vi "DDemo6_-G3.vi"() -> ()   [LabVIEW 2019]
uses:
  uStat400/DropSens uStat400 vis/Parameters.ctl
  uStat400/DropSens uStat400 vis/Serial - Settings mod.ctl
panel:
  out "position":bool
  out "main":bool
  out "graphs":bool
  out "potentiostat":bool
  in  "XI/YI":bool
  out "Camera":bool
  out "YV Graph":cluster{"X array":dbl[], "y array":dbl[]}(graph)
  out "XV Graph":cluster{"X array":dbl[], "y array":dbl[]}(graph)
  out "Iarray":dbl[](array[numeric])
  out "Yarray":dbl[](array[numeric])
  out "Xarray":dbl[](array[numeric])
  out "Moving":i32
  out "Status":bool
  out "error out":errorcluster
  out "Curves":cluster{dbl[], dbl[]}[](array[cluster])=[{[0.1, 0.102, 0.104, 0.106, 0.108, 0.11, 0.112, 0.114, 0.116, 0.118, 0.12, 0.122, 0.124, 0.126, 0.128, 0.13, 0.132, 0.134, 0.136, 0.138, 0.14, 0.142, 0.144, 0.146, 0.148, 0.15, 0.152, 0.154, 0.156, 0.158, 0.16, 0.162, 0.164, 0.166, 0.168, 0.17, 0.172, 0.174, 0.176, 0.178, 0.18, 0.182, 0.184, 0.186, 0.188, 0.19, 0.192, 0.194, 0.196, 0.198, 0.2, 0.202, 0.204, 0.206, 0.208, 0.21, 0.212, 0.214, 0.216, 0.218, 0.22, 0.222, 0.224, 0.226, 0.228, 0.23, 0.232, 0.234, 0.236, 0.238, 0.24, 0.242, 0.244, 0.246, 0.248, 0.25, 0.252, 0.254, 0.256, 0.258, 0.26, 0.262, 0.264, 0.266, 0.268, 0.27, 0.272, 0.274, 0.276, 0.278, 0.28, 0.282, 0.284, 0.286, 0.288, 0.29, 0.292, 0.294, 0.296, 0.298, 0.3, 0.302, 0.304, 0.306, 0.308, 0.31, 0.312, 0.314, 0.316, 0.318, 0.32, 0.322, 0.324, 0.326, 0.328, 0.33, 0.332, 0.334, 0.336, 0.338, 0.34, 0.342, 0.344, 0.346, 0.348, 0.35, 0.352, 0.354, 0.356, 0.358, 0.36, 0.362, 0.364, 0.366, 0.368, 0.37, 0.372, 0.374, 0.376, 0.378, 0.38, 0.382, 0.384, 0.386, 0.388, 0.39, 0.392, 0.394, 0.396, 0.398, 0.4, 0.402, 0.404, 0.406, 0.408, 0.41, 0.412, 0.414, 0.416, 0.418, 0.42, 0.422, 0.424, 0.426, 0.428, 0.43, 0.432, 0.434, 0.436, 0.438, 0.44, 0.442, 0.444, 0.446, 0.448, 0.45, 0.452, 0.454, 0.456, 0.458, 0.46, 0.462, 0.464, 0.466, 0.468, 0.47, 0.472, 0.474, 0.476, 0.478, 0.48, 0.482, 0.484, 0.486, 0.488, 0.49, 0.492, 0.494, 0.496, 0.498, 0.5, 0.502, 0.504, 0.506, 0.508, 0.51, 0.512, 0.514, 0.516, 0.518, 0.52, 0.522, 0.524, 0.526, 0.528, 0.53, 0.532, 0.534, 0.536, 0.538, 0.54, 0.542, 0.544, 0.546, 0.548, 0.55, 0.552, 0.554, 0.556, 0.558, 0.56, 0.562, 0.564, 0.566, 0.568, 0.57, 0.572, 0.574, 0.576, 0.578, 0.58, 0.582, 0.584, 0.586, 0.588, 0.59, 0.592, 0.594, 0.596, 0.598, 0.6, 0.602, 0.604, 0.606, 0.608, 0.61, 0.612, 0.614, 0.616, 0.618, 0.62, 0.622, 0.624, 0.626, 0.628, 0.63, 0.632, 0.634, 0.636, 0.638, 0.64, 0.642, 0.644, 0.646, 0.648, 0.65, 0.652, 0.654, 0.656, 0.658, 0.66, 0.662, 0.664, 0.666, 0.668, 0.67, 0.672, 0.674, 0.676, 0.678, 0.68, 0.682, 0.684, 0.686, 0.688, 0.69, 0.692, 0.694, 0.696, 0.698, 0.7, 0.702, 0.704, 0.706, 0.708, 0.71, 0.712, 0.714, 0.716, 0.718, 0.72, 0.722, 0.724, 0.726, 0.728, 0.73, 0.732, 0.734, 0.736, 0.738, 0.74, 0.742, 0.744, 0.746, 0.748, 0.75, 0.752, 0.754, 0.756, 0.758, 0.76, 0.762, 0.764, 0.766, 0.768, 0.77, 0.772, 0.774, 0.776, 0.778, 0.78, 0.782, 0.784, 0.786, 0.788, 0.79, 0.792, 0.794, 0.796, 0.798, 0.8, 0.802, 0.804, 0.806, 0.808, 0.81, 0.812, 0.814, 0.816, 0.818, 0.82, 0.822, 0.824, 0.826, 0.828, 0.83, 0.832, 0.834, 0.836, 0.838, 0.84, 0.842, 0.844, 0.846, 0.848, 0.85, 0.852, 0.854, 0.856, 0.858, 0.86, 0.862, 0.864, 0.866, 0.868, 0.87, 0.872, 0.874, 0.876, 0.878, 0.88, 0.882, 0.884, 0.886, 0.888, 0.89, 0.892, 0.894, 0.896, 0.898, 0.9], [5e-05, 6.25e-05, 5e-05, 6.25e-05, 5e-05, 5e-05, 5e-05, 7.5e-05, 5e-05, 6.25e-05, 5e-05, 6.25e-05, 5e-05, 6.25e-05, 5e-05, 6.25e-05, 5e-05, 6.25e-05, 5e-05, 6.25e-05, 5e-05, 6.25e-05, 5e-05, 6.25e-05, 5e-05, 6.25e-05, 5e-05, 6.25e-05, 3.75e-05, 7.5e-05, 5e-05, 6.25e-05, 5e-05, 6.25e-05, 5e-05, 6.25e-05, 5e-05, 6.25e-05, 5e-05, 6.25e-05, 5e-05, 7.5e-05, 5e-05, 6.25e-05, 5e-05, 6.25e-05, 5e-05, 7.5e-05, 6.25e-05, 6.25e-05, 5e-05, 6.25e-05, 5e-05, 7.5e-05, 5e-05, 6.25e-05, 5e-05, 6.25e-05, 5e-05, 6.25e-05, 5e-05, 6.25e-05, 5e-05, 7.5e-05, 5e-05, 6.25e-05, 5e-05, 7.5e-05, 6.25e-05, 6.25e-05, 5e-05, 6.25e-05, 5e-05, 6.25e-05, 5e-05, 6.25e-05, 5e-05, 6.25e-05, 5e-05, 6.25e-05, 5e-05, 6.25e-05, 5e-05, 6.25e-05, 5e-05, 6.25e-05, 5e-05, 6.25e-05, 5e-05, 6.25e-05, 5e-05, 6.25e-05, 5e-05, 6.25e-05, 5e-05, 6.25e-05, 5e-05, 6.25e-05, 3.75e-05, 6.25e-05, 5e-05, 6.25e-05, 5e-05, 6.25e-05, 5e-05, 6.25e-05, 5e-05, 6.25e-05, 5e-05, 6.25e-05, 5e-05, 6.25e-05, 5e-05, 6.25e-05, 5e-05, 7.5e-05, 5e-05, 7.5e-05, 5e-05, 6.25e-05, 5e-05, 6.25e-05, 5e-05, 7.5e-05, 3.75e-05, 6.25e-05, 5e-05, 7.5e-05, 5e-05, 7.5e-05, 3.75e-05, 7.5e-05, 5e-05, 6.25e-05, 5e-05, 7.5e-05, 5e-05, 6.25e-05, 5e-05, 7.5e-05, 3.75e-05, 7.5e-05, 5e-05, 6.25e-05, 5e-05, 6.25e-05, 5e-05, 6.25e-05, 5e-05, 7.5e-05, 3.75e-05, 7.5e-05, 3.75e-05, 6.25e-05, 5e-05, 6.25e-05, 5e-05, 7.5e-05, 3.75e-05, 6.25e-05, 5e-05, 6.25e-05, 5e-05, 6.25e-05, 3.75e-05, 7.5e-05, 5e-05, 7.5e-05, 3.75e-05, 6.25e-05, 5e-05, 6.25e-05, 3.75e-05, 6.25e-05, 5e-05, 6.25e-05, 5e-05, 6.25e-05, 5e-05, 6.25e-05, 5e-05, 7.5e-05, 5e-05, 7.5e-05, 5e-05, 6.25e-05, 5e-05, 7.5e-05, 5e-05, 7.5e-05, 5e-05, 7.5e-05, 5e-05, 7.5e-05, 5e-05, 7.5e-05, 5e-05, 7.5e-05, 6.25e-05, 8.75e-05, 6.25e-05, 7.5e-05, 5e-05, 7.5e-05, 5e-05, 7.5e-05, 5e-05, 7.5e-05, 6.25e-05, 7.5e-05, 5e-05, 7.5e-05, 5e-05, 7.5e-05, 5e-05, 7.5e-05, 5e-05, 7.5e-05, 5e-05, 6.25e-05, 5e-05, 7.5e-05, 5e-05, 7.5e-05, 5e-05, 6.25e-05, 5e-05, 7.5e-05, 3.75e-05, 6.25e-05, 3.75e-05, 6.25e-05, 3.75e-05, 6.25e-05, 3.75e-05, 6.25e-05, 5e-05, 7.5e-05, 5e-05, 7.5e-05, 5e-05, 7.5e-05, 3.75e-05, 7.5e-05, 5e-05, 7.5e-05, 5e-05, 6.25e-05, 3.75e-05, 6.25e-05, 5e-05, 6.25e-05, 3.75e-05, 7.5e-05, 5e-05, 6.25e-05, 3.75e-05, 6.25e-05, 5e-05, 6.25e-05, 5e-05, 6.25e-05, 5e-05, 7.5e-05, 3.75e-05, 6.25e-05, 5e-05, 6.25e-05, 3.75e-05, 7.5e-05, 5e-05, 6.25e-05, 5e-05, 6.25e-05, 5e-05, 6.25e-05, 5e-05, 6.25e-05, 5e-05, 6.25e-05, 5e-05, 6.25e-05, 3.75e-05, 6.25e-05, 5e-05, 6.25e-05, 5e-05, 7.5e-05, 5e-05, 6.25e-05, 5e-05, 6.25e-05, 5e-05, 6.25e-05, 5e-05, 6.25e-05, 5e-05, 6.25e-05, 3.75e-05, 6.25e-05, 3.75e-05, 6.25e-05, 5e-05, 6.25e-05, 3.75e-05, 6.25e-05, 3.75e-05, 6.25e-05, 5e-05, 6.25e-05, 5e-05, 6.25e-05, 5e-05, 6.25e-05, 5e-05, 6.25e-05, 5e-05, 6.25e-05, 5e-05, 7.5e-05, 5e-05, 6.25e-05, 3.75e-05, 6.25e-05, 5e-05, 7.5e-05, 5e-05, 7.5e-05, 5e-05, 6.25e-05, 5e-05, 7.5e-05, 3.75e-05, 6.25e-05, 5e-05, 7.5e-05, 5e-05, 6.25e-05, 5e-05, 6.25e-05, 5e-05, 7.5e-05, 3.75e-05, 6.25e-05, 5e-05, 6.25e-05, 5e-05, 7.5e-05, 5e-05, 6.25e-05, 5e-05, 6.25e-05, 3.75e-05, 6.25e-05, 3.75e-05, 6.25e-05, 3.75e-05, 7.5e-05, 3.75e-05, 6.25e-05, 5e-05, 6.25e-05, 3.75e-05, 6.25e-05, 3.75e-05, 6.25e-05, 5e-05, 7.5e-05, 5e-05, 6.25e-05, 5e-05, 6.25e-05, 3.75e-05, 6.25e-05, 3.75e-05, 6.25e-05, 5e-05, 5e-05, 3.75e-05, 6.25e-05, 5e-05, 6.25e-05, 3.75e-05, 6.25e-05, 3.75e-05, 6.25e-05, 5e-05, 6.25e-05, 3.75e-05, 6.25e-05, 3.75e-05, 7.5e-05, 3.75e-05, 6.25e-05, 5e-05, 6.25e-05, 5e-05, 6.25e-05, 5e-05, 6.25e-05, 5e-05]}, ...(4 in all)]
  in  "Serial Settings":T1={"baud rate"=115200, "data bits"=8, "parity"=enum."None", "stop bits"=10, "flow control"=0} {"flow control" items=["None"=0, "XON/XOFF"=1, "RTS/CTS"=2, "DTR/DSR"=4]; "stop bits" items=["1.0"=10, "1.5"=15, "2.0"=20]; "data bits" min=5 max=8 step=1; "baud rate" items=["75"=75, "110"=110, "134"=134, "150"=150, "300"=300, "600"=600, "1200"=1200, "1800"=1800, "2400"=2400, "4800"=4800, "7200"=7200, "9600"=9600, "14400"=14400, "19200"=19200, "28800"=28800, "38400"=38400, "56000"=56000, "57600"=57600, "115200"=115200, "128000"=128000, "230400"=230400]}
  in  "Node list":string[](tree)=["Node 1 - Ch1"]
  in  "Cluster 5":T3={"Parameters M"=[{"Param"="Estep [V]", "Values"=0.002}, {"Param"="Srate [V/s]", "Values"=0.05}], "Parameters N 8"=[], "Parameters N 7"=[], "Parameters N 6"=[], "Parameters N 5"=[{"Param"="Ebegin [V]", "Values"=0.1}, {"Param"="Eend [V]", "Values"=0.9}, {"Param"="Estep [V]", "Values"=0.002}, {"Param"="Srate [V/s]", "Values"=0.05}], "Parameters N 4"=[{"Param"="Ebegin [V]", "Values"=0.1}, {"Param"="Eend [V]", "Values"=0.9}], "Parameters N 3"=[{"Param"="Ebegin [V]", "Values"=0.1}, {"Param"="Eend [V]", "Values"=0.9}], "Parameters N 2"=[{"Param"="Ebegin [V]", "Values"=0.1}, {"Param"="Eend [V]", "Values"=0.9}], "Parameters N 1"=[{"Param"="Ebegin [V]", "Values"=0.1}, {"Param"="Eend [V]", "Values"=0.9}, {"Param"="Estep [V]", "Values"=0.002}, {"Param"="Srate [V/s]", "Values"=0.05}]}
  in  "Cluster 4":T4={"Pretr M"=[{"Param"="Econd [V]", "Values"=0.0}, {"Param"="Tcond [s]", "Values"=0.0}, {"Param"="Edep [V]", "Values"=0.0}, {"Param"="Tdep [s]", "Values"=0.0}, {"Param"="Tequil [s]", "Values"=3.0}], "Pretr N 7"=[{"Param"="Econd [V]", "Values"=0.0}, {"Param"="Tcond [s]", "Values"=0.0}, {"Param"="Edep [V]", "Values"=0.0}, {"Param"="Tdep [s]", "Values"=0.0}, {"Param"="Tequil [s]", "Values"=3.0}], "Pretr N 5"=[{"Param"="Econd [V]", "Values"=0.0}, {"Param"="Tcond [s]", "Values"=0.0}, {"Param"="Edep [V]", "Values"=0.0}, {"Param"="Tdep [s]", "Values"=0.0}, {"Param"="Tequil [s]", "Values"=3.0}], "Pretr N 4"=[{"Param"="Econd [V]", "Values"=0.0}, {"Param"="Tcond [s]", "Values"=0.0}, {"Param"="Edep [V]", "Values"=0.0}, {"Param"="Tdep [s]", "Values"=0.0}, {"Param"="Tequil [s]", "Values"=3.0}], "Pretr N 3"=[{"Param"="Econd [V]", "Values"=0.0}, {"Param"="Tcond [s]", "Values"=0.0}, {"Param"="Edep [V]", "Values"=0.0}, {"Param"="Tdep [s]", "Values"=0.0}, {"Param"="Tequil [s]", "Values"=3.0}], "Pretr N 2"=[{"Param"="Econd [V]", "Values"=0.0}, {"Param"="Tcond [s]", "Values"=0.0}, {"Param"="Edep [V]", "Values"=0.0}, {"Param"="Tdep [s]", "Values"=0.0}, {"Param"="Tequil [s]", "Values"=3.0}], "Pretr N 1"=[{"Param"="Econd [V]", "Values"=0.0}, {"Param"="Tcond [s]", "Values"=0.0}, {"Param"="Edep [V]", "Values"=0.0}, {"Param"="Tdep [s]", "Values"=0.0}, {"Param"="Tequil [s]", "Values"=3.0}], "Pretr N 8"=[{"Param"="Econd [V]", "Values"=0.0}, {"Param"="Tcond [s]", "Values"=0.0}, {"Param"="Edep [V]", "Values"=0.0}, {"Param"="Tdep [s]", "Values"=0.0}, {"Param"="Tequil [s]", "Values"=3.0}], "Pretr N 6"=[{"Param"="Econd [V]", "Values"=0.0}, {"Param"="Tcond [s]", "Values"=0.0}, {"Param"="Edep [V]", "Values"=0.0}, {"Param"="Tdep [s]", "Values"=0.0}, {"Param"="Tequil [s]", "Values"=3.0}]}
  in  "Cluster 3":T5 {"Option N 1"."StandbyPot" format="%.3g"; "Option N 2"."StandbyPot" format="%.3g"; "Option N 4"."StandbyPot" format="%.3g"; "Option N 6"."StandbyPot" format="%.3g"; "Option N 7"."StandbyPot" format="%.3g"; "Option N 8"."StandbyPot" format="%.3g"; "Option N 3"."StandbyPot" format="%.3g"; "Option N 5"."StandbyPot" format="%.3g"; "Option M"."StandbyPot" format="%.3g"}
  in  "Cluster 2":T6
  out "Cluster":T7={"Technique M"="Linear Sweep Voltammetry", "Technique N 8"="Linear Sweep Voltammetry", "Technique N 7"="Linear Sweep Voltammetry", "Technique N 6"="Linear Sweep Voltammetry", "Technique N 5"="Linear Sweep Voltammetry", "Technique N 4"="Linear Sweep Voltammetry", "Technique N 3"="Linear Sweep Voltammetry", "Technique N 2"="Linear Sweep Voltammetry", "Technique N 1"="Linear Sweep Voltammetry"}
  in  "XYXA":bool
  out "Image Out":T8(plugin-control)
  out "ArAy":string[](array[string])
  out "ArAx":string[](array[string])
  out "Rel_act_pos":string
  out "True A":dbl format="%#.3g"
  out "True Z":dbl format="%#.3f"
  out "True Y":dbl format="%#.3f"
  out "True X":dbl format="%#.3f"
  out "MDI":string
  in  "Tab Control":T9(tab)
  in  "Copy current position":bool
  in  "Stop all":bool
  in  "Move":bool
  in  "A":dbl
  in  "Z":dbl
  in  "Y":dbl
  in  "X":dbl
  in  "Home":bool
  out "Sent value":string
  in  "A-":bool
  in  "A+":bool
  in  "stop step":bool
  in  "z-":bool
  in  "z+":bool
  out "Step":bool
  out "Jog":bool=TRUE
  in  "Step size (mm)":dbl
  in  "Jog?":bool=TRUE
  in  "Speed (mm/s) manual":dbl(knob)=10.0 min=1.0 max=500.0 step=1.0 scale=1.0..500.0 scale format="%#_6f"
  in  "y-":bool
  in  "y+":bool
  in  "x-":bool
  in  "x+":bool
  out "manual":bool
  in  "2D stop":bool
  in  "Wait (ms)":dbl=1.0 min=1.0 step=1.0
  in  "Speed (micron/s) 2D":dbl(knob)=1.0 min=1.0 max=500.0 step=1.0 scale=1.0..500.0 scale format="%#_6f"
  in  "2D start":bool
  in  "No. of teps":dbl=1.0 min=1.0 step=1.0
  in  "Y1":dbl step=0.0001 format="%#.3f"
  in  "Y0":dbl step=0.0001 format="%#.3f"
  in  "X1":dbl step=0.001 format="%#.3f"
  in  "X0":dbl step=0.001 format="%#.3f"
  in  "Stop A":bool
  out "String":string
  in  "Speed (micron/s) A":dbl(knob)=1.0 min=1.0 max=500.0 step=1.0 scale=1.0..500.0 scale format="%#_6f"
  in  "y0":dbl min=0.0 step=0.001 format="%#.3f"
  in  "x0":dbl min=0.0 step=0.001 format="%#.3f"
  in  "x1":dbl min=0.0 step=0.001 format="%#.3f"
  in  "y1":dbl min=0.0 step=0.001 format="%#.3f"
  in  "Line displacement":dbl=0.001 min=0.001 step=0.001 format="%#_3f"
  in  "Step size":dbl=0.001 min=0.001 step=0.001 format="%#_3f"
  in  "Area start":bool
  in  "Wait (ms) Area":dbl=1000.0 min=1.0 step=1.0
  out "Status":bool
  out "Actual I/U 2":dbl
  out "Config Status":u8(slide)=73 scale=0.0..66.0
  out "Actual Values":T10 {"Actual I/U" format="%#_6f"}
  in  "VISA resource name":refnum<visa-resource-name>="COM5"
  in  "Check port":bool
  in  "stop Measuring":bool
  out "result":bool
  # "Target position"
  # "Start"
  # "Finish"
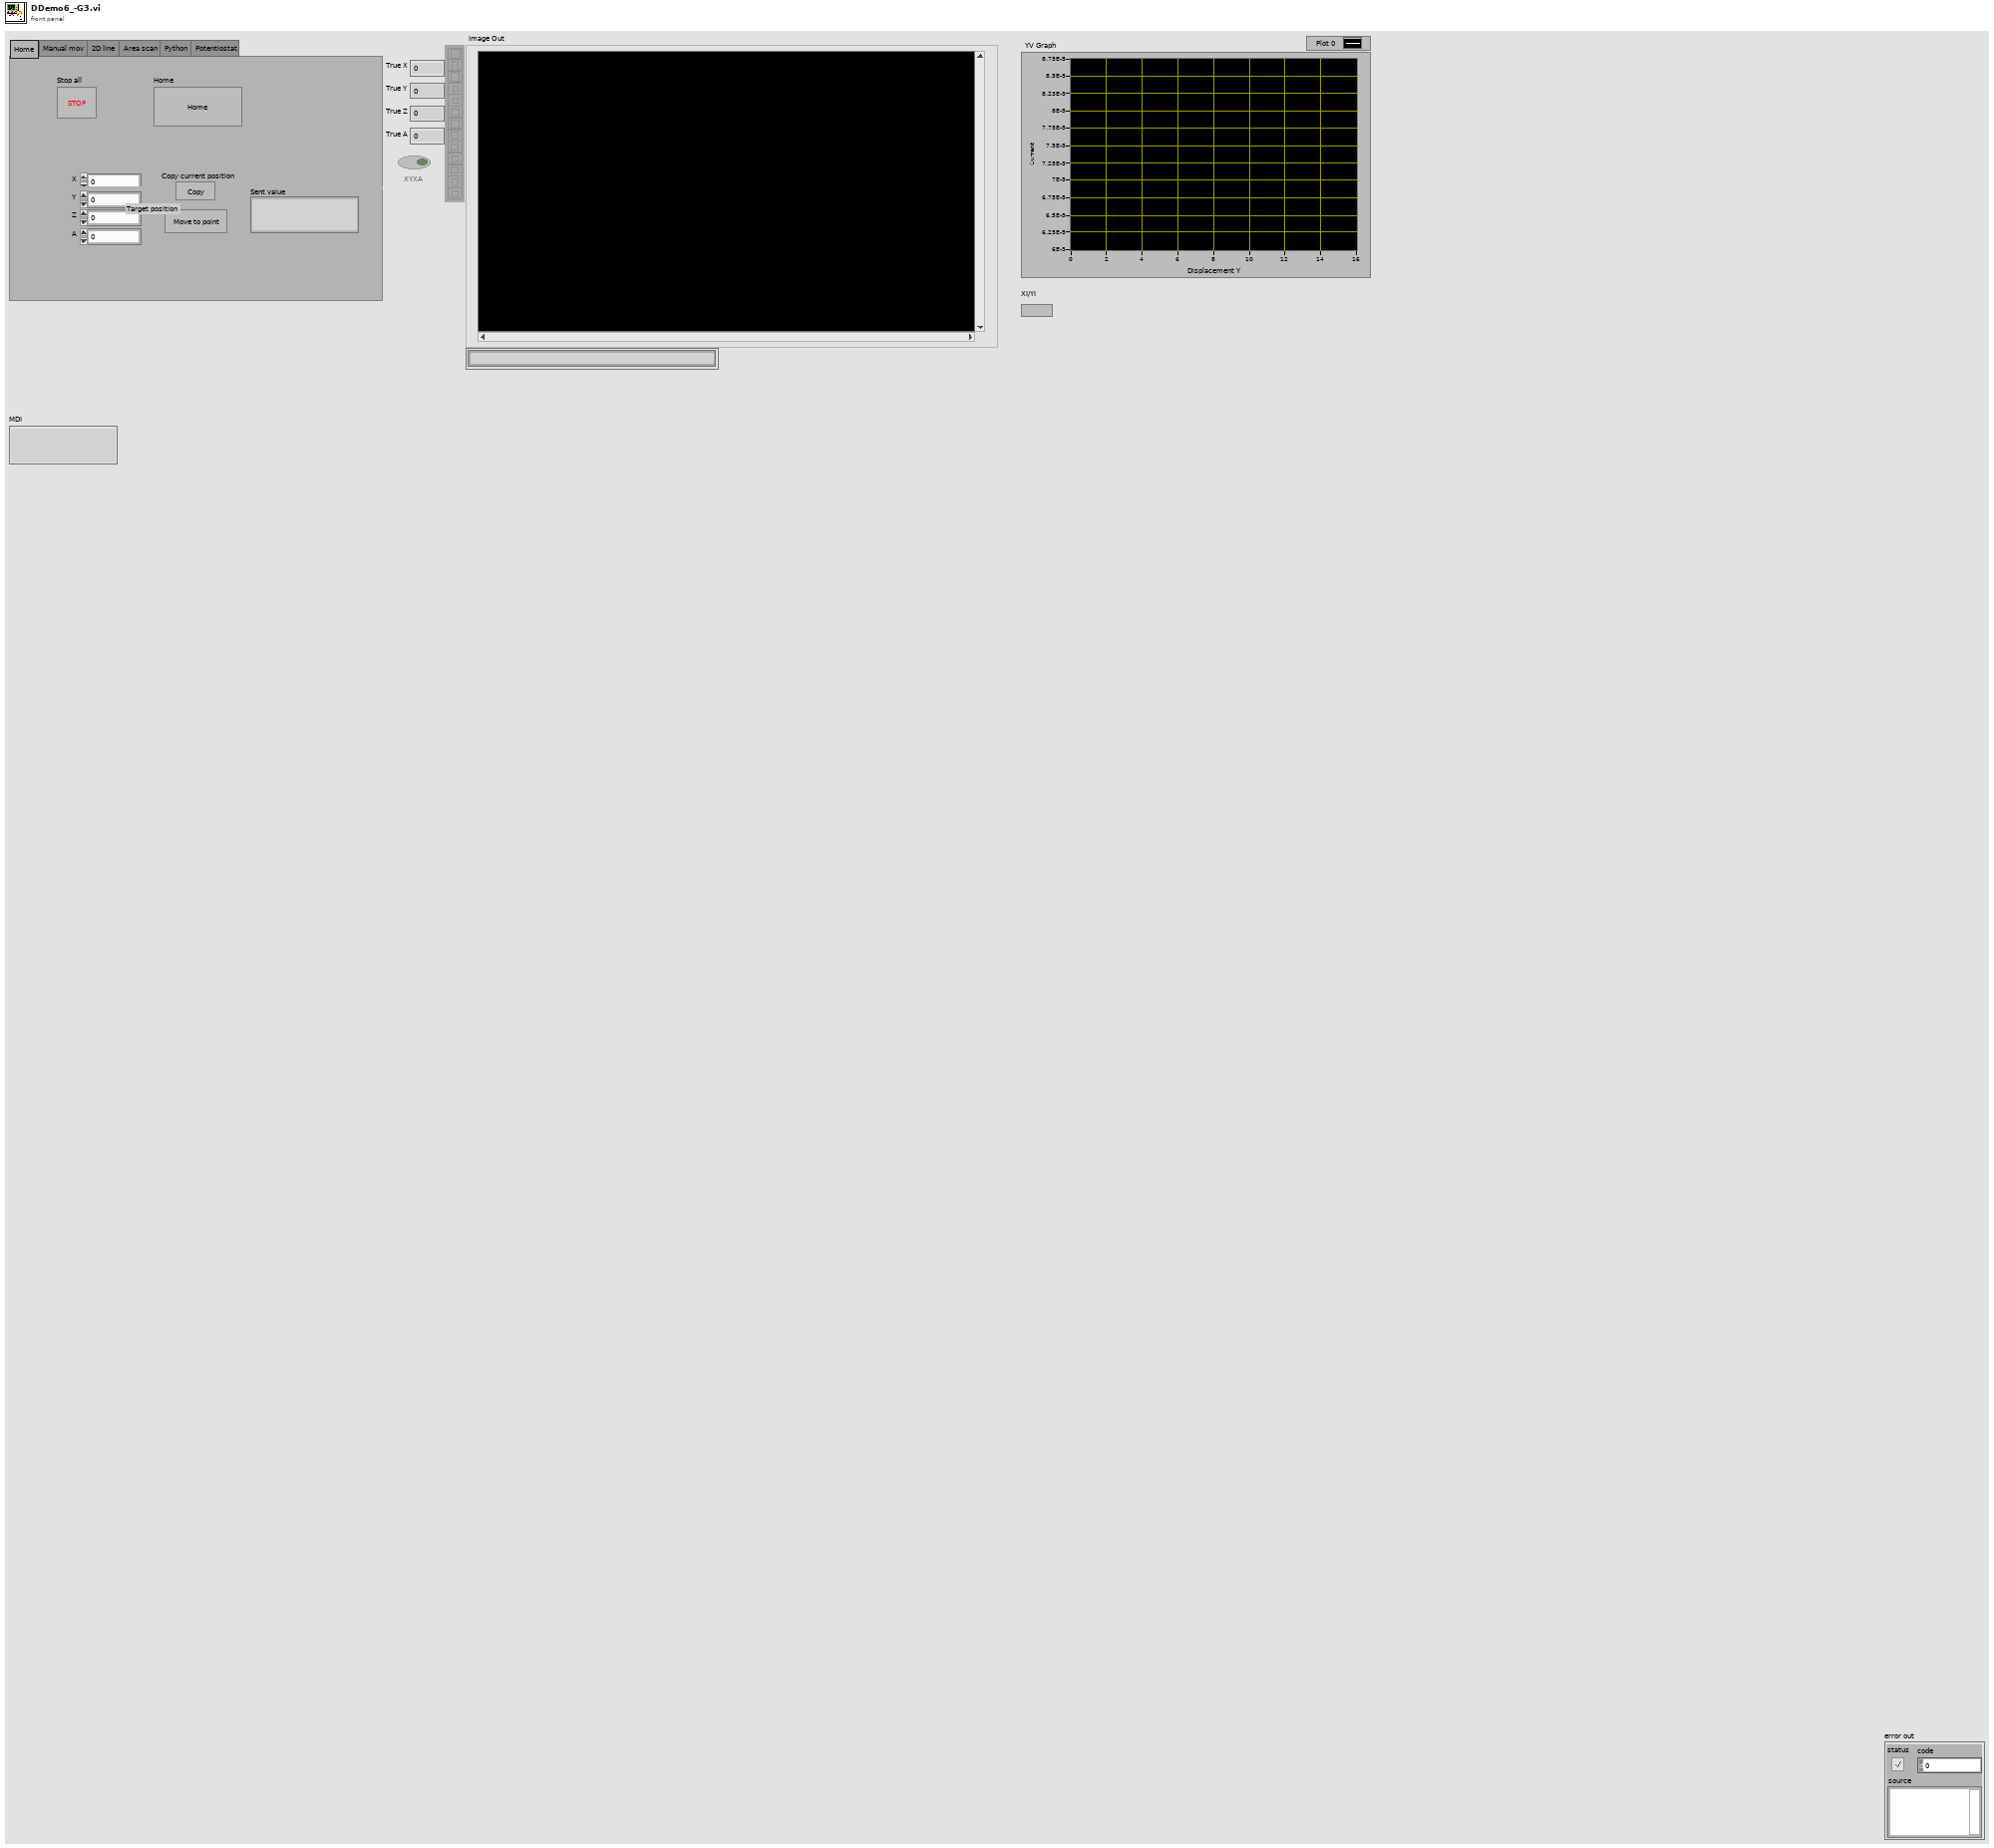
[diagram p1: front panel]
types:
  T1 = typedef "Serial - Settings mod.ctl" = cluster{"baud rate":u32, "data bits":u16, "parity":enum16{"None", "Odd", "Even", "Mark", "Space"}, "stop bits":u16, "flow control":u16}
  T2 = typedef "Parameters.ctl" = cluster{"Param":string, "Values":dbl}[]
  T3 = cluster{"Parameters M":T2, "Parameters N 8":T2, "Parameters N 7":T2, "Parameters N 6":T2, "Parameters N 5":T2, "Parameters N 4":T2, "Parameters N 3":T2, "Parameters N 2":T2, "Parameters N 1":T2}
  T4 = cluster{"Pretr M":T2, "Pretr N 7":T2, "Pretr N 5":T2, "Pretr N 4":T2, "Pretr N 3":T2, "Pretr N 2":T2, "Pretr N 1":T2, "Pretr N 8":T2, "Pretr N 6":T2}
  T5 = cluster{"Option M":cluster{"Cells":enum32{"No Selection", "Leave cell on", "Standby potential"}, "StandbyPot":dbl}, "Option N 5":cluster{"Cells":enum32{"No Selection", "Leave cell on", "Standby potential"}, "StandbyPot":dbl}, "Option N 3":cluster{"Cells":enum32{"No Selection", "Leave cell on", "Standby potential"}, "StandbyPot":dbl}, "Option N 8":cluster{"Cells":enum32{"No Selection", "Leave cell on", "Standby potential"}, "StandbyPot":dbl}, "Option N 7":cluster{"Cells":enum32{"No Selection", "Leave cell on", "Standby potential"}, "StandbyPot":dbl}, "Option N 6":cluster{"Cells":enum32{"No Selection", "Leave cell on", "Standby potential"}, "StandbyPot":dbl}, "Option N 4":cluster{"Cells":enum32{"No Selection", "Leave cell on", "Standby potential"}, "StandbyPot":dbl}, "Option N 2":cluster{"Cells":enum32{"No Selection", "Leave cell on", "Standby potential"}, "StandbyPot":dbl}, "Option N 1":cluster{"Cells":enum32{"No Selection", "Leave cell on", "Standby potential"}, "StandbyPot":dbl}}
  T6 = cluster{"CR N 8":enum16{"Auto", "10 mA", "1 mA", "100 uA", "10 uA", "1 uA", "100 nA", "10 nA", "1 nA"}, "CR N 7":enum16{"Auto", "10 mA", "1 mA", "100 uA", "10 uA", "1 uA", "100 nA", "10 nA", "1 nA"}, "CR N 6":enum16{"Auto", "10 mA", "1 mA", "100 uA", "10 uA", "1 uA", "100 nA", "10 nA", "1 nA"}, "CR N 5":enum16{"Auto", "10 mA", "1 mA", "100 uA", "10 uA", "1 uA", "100 nA", "10 nA", "1 nA"}, "CR N 4":enum16{"Auto", "10 mA", "1 mA", "100 uA", "10 uA", "1 uA", "100 nA", "10 nA", "1 nA"}, "CR N 3":enum16{"Auto", "10 mA", "1 mA", "100 uA", "10 uA", "1 uA", "100 nA", "10 nA", "1 nA"}, "CR N 2":enum16{"Auto", "10 mA", "1 mA", "100 uA", "10 uA", "1 uA", "100 nA", "10 nA", "1 nA"}, "CR N 1":enum16{"Auto", "10 mA", "1 mA", "100 uA", "10 uA", "1 uA", "100 nA", "10 nA", "1 nA"}}
  T7 = cluster{"Technique M":string, "Technique N 8":string, "Technique N 7":string, "Technique N 6":string, "Technique N 5":string, "Technique N 4":string, "Technique N 3":string, "Technique N 2":string, "Technique N 1":string}
  T8 = typedef "IMAQ Image.ctl" = refnum<image>
  T9 = enum32{"Home", "Manual mov", "2D line", "Area scan", "Python", "Potentiostat"}
  T10 = cluster{"Actual I/U":dbl, "Actual V/T":dbl, "No of Ch":i16}
  T11 = enum16{"Main", "Line", "Area Move", "Enable all", "Move to target", "Get Values"}
  T12 = typedef "Comunication.ctl" = cluster{"VISA resource name out":refnum<visa-resource-name>, "Techniques":T13[], "Tree 2":refnum<vi>, "Nodes":i32[], "Radio Buttons":enum32{"M 1x8", "M 8x1"}, "queue ref":refnum<queue>}
  T13 = typedef "Techniques.ctl" = enum16{"Linear Sweep Voltammetry", "Cyclic Voltammetry", "Square Wave Voltammetry", "Differential Pulse Voltammetry", "Normal Pulse Voltammetry", "Normal Dif. Pulse Voltametry", "AC Voltametry", "Linear Polarization Resistance", "LSV+AD", "CV+AD", "Amperometric Detection", "Zero Resistance Amperometry", "Fast Amperometry", "Pulsed Amperometric Detection", "Multipulsed Amperometric Detection", "Coulometric Detection", "Linear Sweep Potentiometry", "Cyclic Potentiometry", "Potentiometric Detection", "Zero Current Potentiometry", "Fast Potentiometry", "Multipulsed Potentiometric Detection", "PSA Faradaic", "PSA Galvanostatic"}
  T14 = enum8{"Enabled", "Disabled", "Disabled and Grayed Out"}
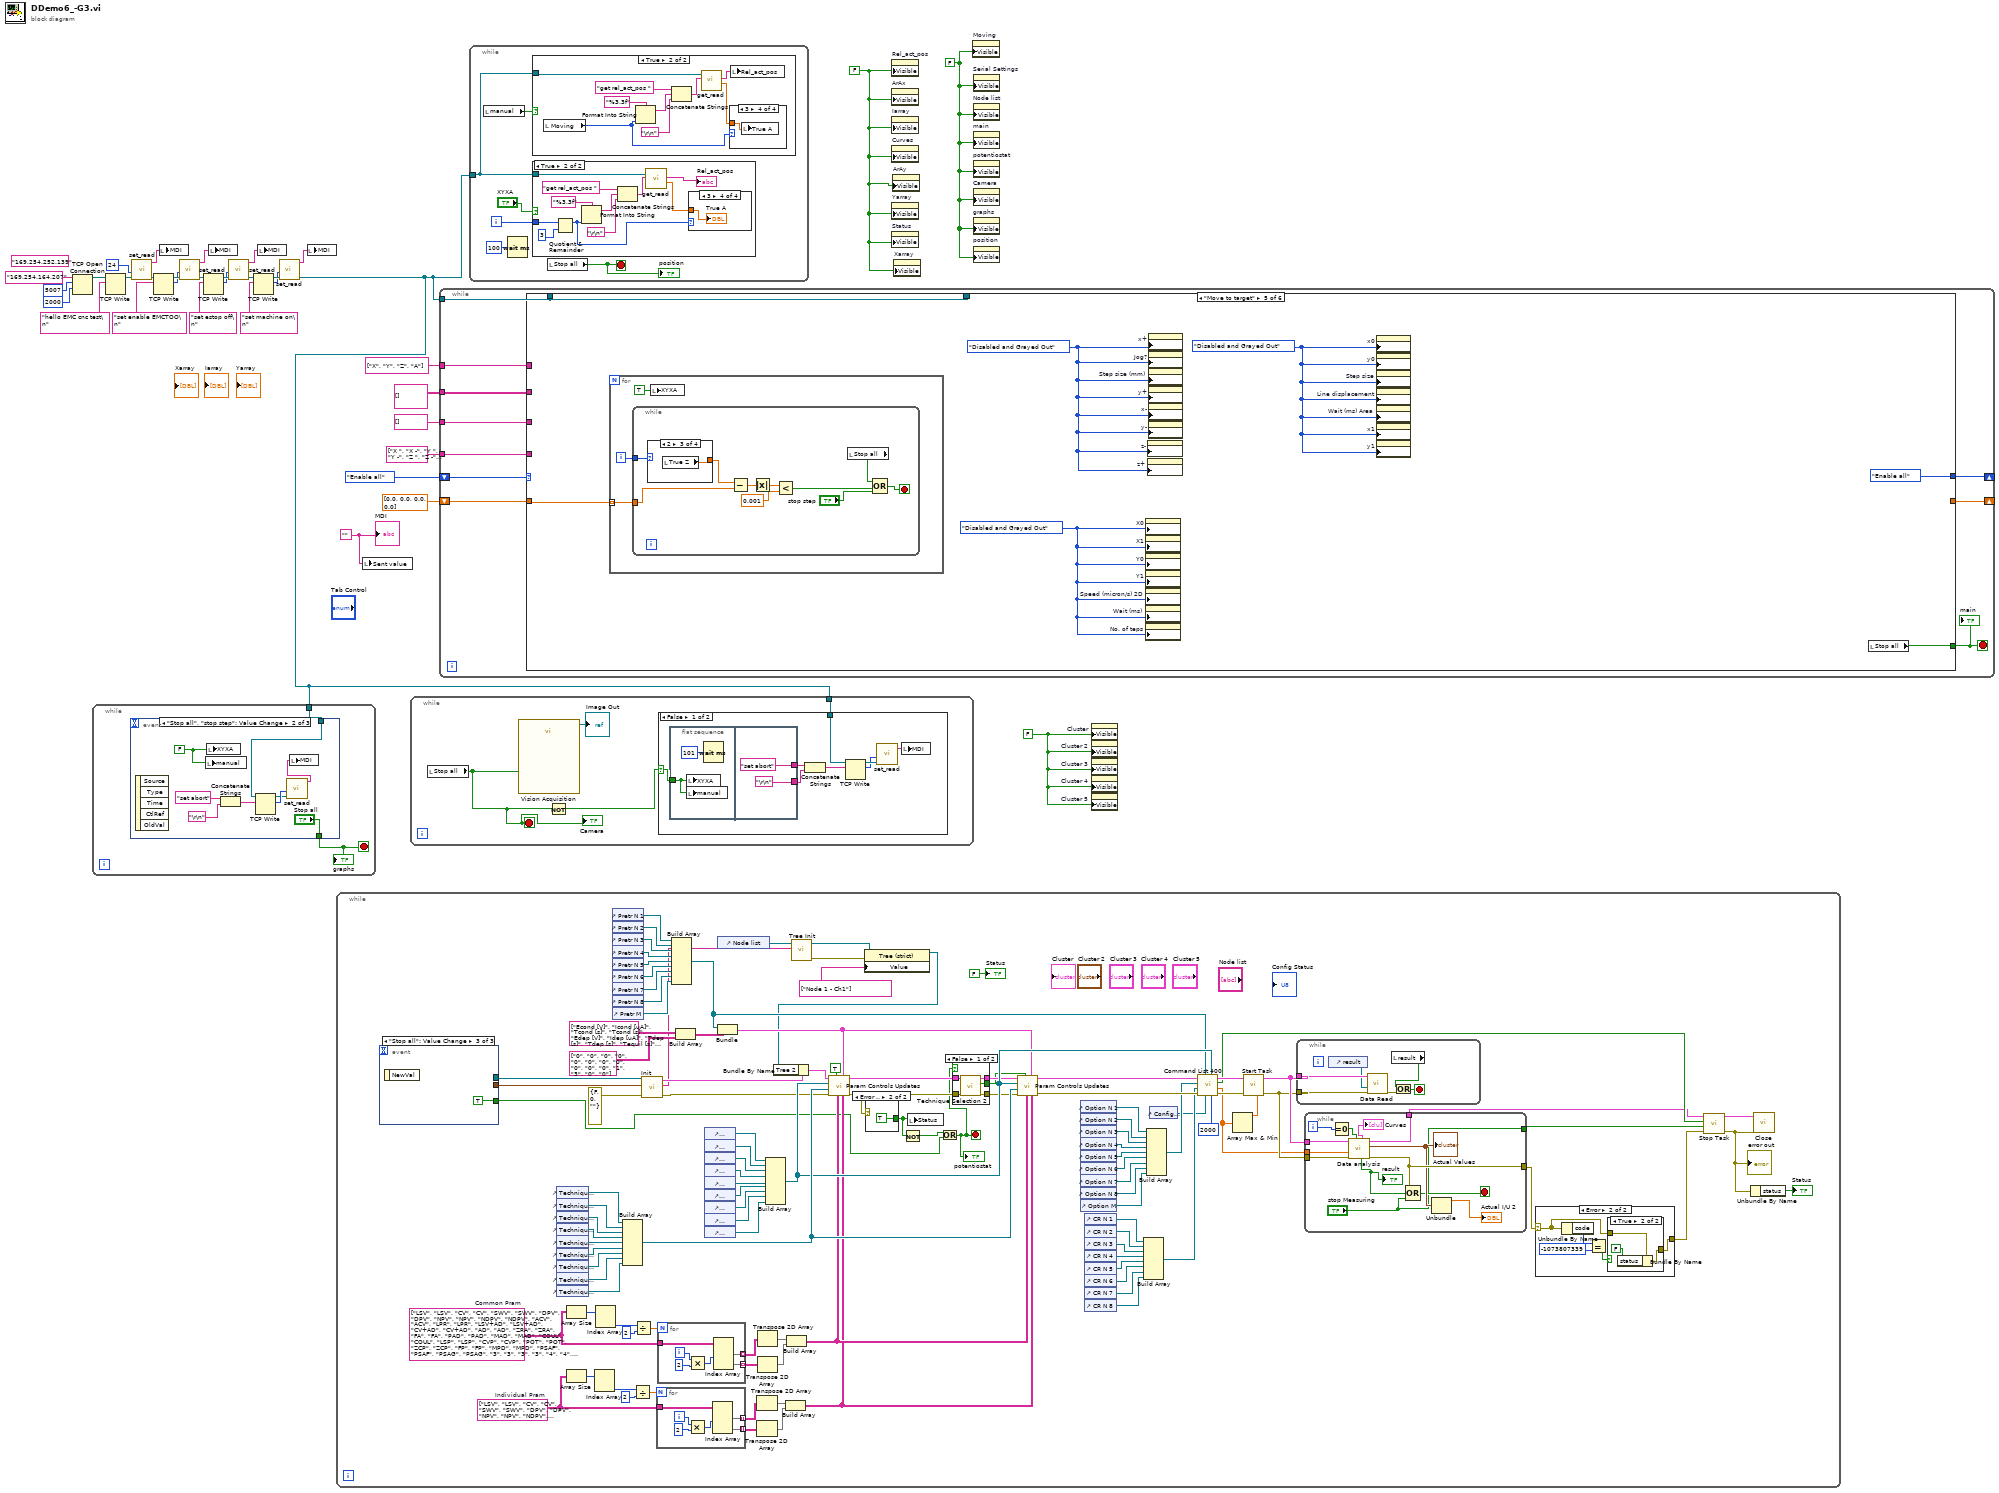
[diagram p0: block diagram]
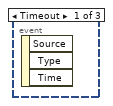
[diagram p3: hidden frame]
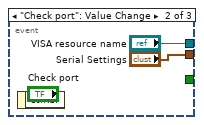
[diagram p4: hidden frame]
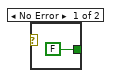
[diagram p5: hidden frame]
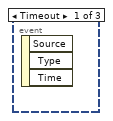
[diagram p8: hidden frame]
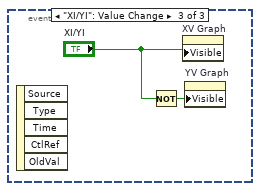
[diagram p9: hidden frame]
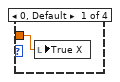
[diagram p12: hidden frame]
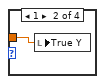
[diagram p13: hidden frame]
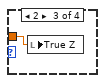
[diagram p14: hidden frame]
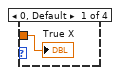
[diagram p16: hidden frame]
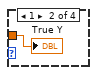
[diagram p17: hidden frame]
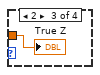
[diagram p18: hidden frame]
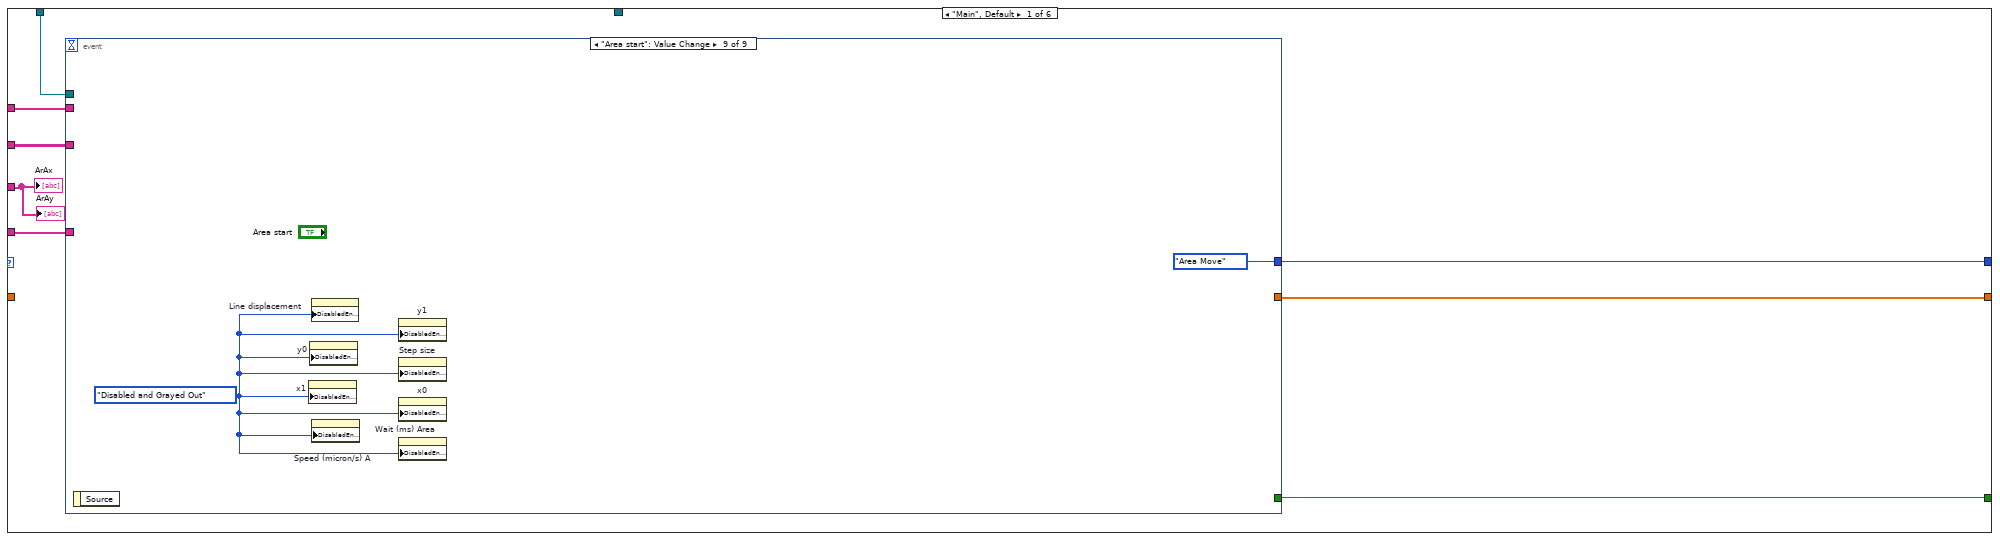
[diagram p19: hidden frame]
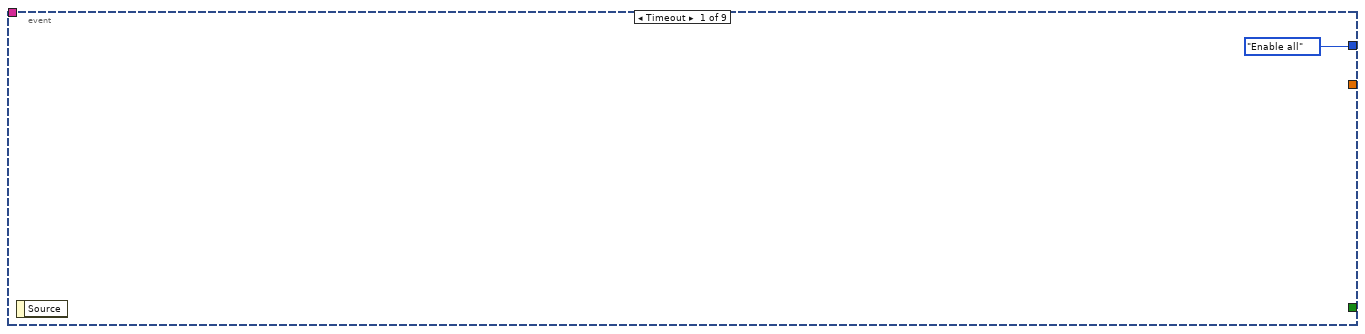
[diagram p20: hidden frame]
diagram:
  w1 = FALSE
  w2 = FALSE
  w5 = FALSE ("Visible")
  (unwired) "169.254.252.139"
  w32 = ""
  n1 = TCP Open Connection(address="169.254.164.207", remote port or service name=5007, timeout ms (60000)=2000) -> (connection ID=w28:refnum<k5>)  [unwired: 2 in, 1 out]
  n2 = TCP Write(connection ID=w28, data in="hello EMC cnc test\n") -> (connection ID out=w27:refnum<k5>)  [unwired: 2 in, 2 out]
  n3 = call "set_read.vi"("connection ID"=w27, "bytes to read"=24) -> ("connection ID 2"=w26:refnum<k5>, "concatenated string"=w13:string)  [unwired: 4 in]
  n4 = TCP Write(connection ID=w26, data in="set enable EMCTOO\n") -> (connection ID out=w25:refnum<k5>, bytes written=w12:i32)  [unwired: 2 in, 1 out]
  n5 = local write "MDI"(w13) -> ()
  n6 = call "set_read.vi"("connection ID"=w25, "bytes to read"=w12) -> ("connection ID 2"=w24:refnum<k5>, "concatenated string"=w16:string)  [unwired: 4 in]
  n7 = TCP Write(connection ID=w24, data in="set estop off\n") -> (connection ID out=w23:refnum<k5>, bytes written=w11:i32)  [unwired: 2 in, 1 out]
  n8 = local write "MDI"(w16) -> ()
  n9 = call "set_read.vi"("connection ID"=w23, "bytes to read"=w11) -> ("connection ID 2"=w22:refnum<k5>, "concatenated string"=w15:string)  [unwired: 4 in]
  n10 = TCP Write(connection ID=w22, data in="set machine on\n") -> (connection ID out=w21:refnum<k5>, bytes written=w10:i32)  [unwired: 2 in, 1 out]
  n11 = local write "MDI"(w15) -> ()
  n12 = call "set_read.vi"("connection ID"=w21, "bytes to read"=w10) -> ("connection ID 2"=w3:refnum<k5>, "concatenated string"=w14:string)  [unwired: 4 in]
  n13 = while {
    tunnel: w3 -> [w36]
    stop <- w35 stop-if-true
    n14 = event shown="[1] \"Stop all\", \"stop step\": Value Change" {
      selector: _ -> [_ _ _]
      dyn-events: _ -> [_ _ _]
      timeout: _ -> [_ _ _]
      tunnel: w36 -> [_ w42 _]
      tunnel: [_ "Stop all" _] -> w35
      event Timeout {
        n15 = event-data() -> ()  [unwired: 1 in, 3 out]
      }
      event "Stop all", "stop step": Value Change {
        w45 = FALSE
        n16 = event-data() -> ()  [unwired: 1 in, 5 out]
        n17 = local write "manual"(w45) -> ()
        n18 = local write "XYXA"(w45) -> ()
        n19 = Concatenate Strings("set abort", "\r\n") -> (w39:string)
        n20 = TCP Write(connection ID=w42, data in=w39) -> (connection ID out=w43:refnum<k5>, bytes written=w44:i32)  [unwired: 2 in, 1 out]
        n21 = call "set_read.vi"("connection ID"=w43, "bytes to read"=w44) -> ("concatenated string"=w38:string)  [unwired: 4 in, 1 out]
        n22 = local write "MDI"(w38) -> ()
      }
      event "XI/YI": Value Change {
        n23 = event-data() -> ()  [unwired: 1 in, 5 out]
        n24 = Not(x="XI/YI") -> (.not. x?=w47:bool)
        n25 = property on="XV Graph" class="XYGraph (strict)"("Visible"="XI/YI") -> ()  [unwired: 2 in, 2 out]
        n26 = property on="YV Graph" class="XYGraph (strict)"("Visible"=w47) -> ()  [unwired: 2 in, 2 out]
      }
    }
    "graphs" <- w35
  }
  n27 = local write "MDI"(w14) -> ()
  n28 = while {
    stop <- w48 stop-if-true
    w58 = string[][] [["LSV", "LSV", "CV", "CV", "SWV", "SWV", "DPV", "DPV", "NPV", "NPV", "NDPV", "NDPV", "ACV", "ACV", "LPR", "LPR", "LSV+AD", "LSV+AD", "CV+AD", "CV+AD", "AD", "AD", "ZRA", "ZRA", "FA", "FA", "PAD", "PAD", "MAD", "MAD", "COUL", "COUL", "LSP", "LSP", "CVP", "CVP", "POT", "POT", "ZCP", "ZCP", "FP", "FP", "MPD", "MPD", "PSAF", "PSAF", "PSAG", "PSAG"], ["2", "2", "3", "3", "2", "2", "2", "2", "2", "2", "2", "2", "2", "2", "2", "2", "0", "0", "0", "0", "1", "1", "0", "0", "1", "1", "1", "1", "8", "8", "1", "1", "2", "2", "3", "3", "1", "1", "0", "0", "1", "1", "8", "8", "0", "0", "0", "0"], ["Ebegin [V]", "0.1", "Ebegin [V]", "0.1", "Ebegin [V]", "0.45", "Ebegin [V]", "0.45", "Ebegin [V]", "0", "Ebegin [V]", "0", "Ebegin [V]", "-0.9", "Ebegin [V]", "-0.1", "", "", "", "", "E [V]", "-0.1", "", "", "E [V]", "-0.1", "Ei [V]", "-0.1", "Steps", "1", "E [V]", "-0.1", "Ibegin [uA]", "0", "Ibegin [uA]", "0.5", "Ibegin [uA]", "-5", "", "", "Ibegin [uA]", "0", "Steps", "1", "", "", "", ""], ["Eend [V]", "0.9", "Evtx1 [V]", "0.9", "Eend [V]", "-0.15", "Eend [V]", "-0.15", "Eend [V]", "0.5", "Eend [V]", "0.5", "Eend [V]", "-0.2", "Eend [V]", "0.1", "", "", "", "", "", "", "", "", "", "", "", "", "Cell off", "1", "", "", "Iend [uA]", "0.5", "Ivtx1 [uA]", "1", "", "", "", "", "", "", "Cell off", "1", "", "", "", ""], ["", "", "Evtx2 [V]", "-0.1", "", "", "", "", "", "", "", "", "", "", "", "", "", "", "", "", "", "", "", "", "", "", "", "", "Limits", "1", "", "", "", "", "Ivtx2 [uA]", "0", "", "", "", "", "", "", "Limits", "1", "", "", "", ""], ["", "", "", "", "", "", "", "", "", "", "", "", "", "", "", "", "", "", "", "", "", "", "", "", "", "", "", "", "Cell 1 [Off/On]", "1", "", "", "", "", "", "", "", "", "", "", "", "", "Cell 1 [Off/On]", "1", "", "", "", ""], ["", "", "", "", "", "", "", "", "", "", "", "", "", "", "", "", "", "", "", "", "", "", "", "", "", "", "", "", "E1 [V]", "0.1", "", "", "", "", "", "", "", "", "", "", "", "", "I1 [uA]", "100", "", "", "", ""], ["", "", "", "", "", "", "", "", "", "", "", "", "", "", "", "", "", "", "", "", "", "", "", "", "", "", "", "", "t1 [s]", "1", "", "", "", "", "", "", "", "", "", "", "", "", "t1 [s]", "1", "", "", "", ""], ["", "", "", "", "", "", "", "", "", "", "", "", "", "", "", "", "", "", "", "", "", "", "", "", "", "", "", "", "Lim1> [uA]", "40000", "", "", "", "", "", "", "", "", "", "", "", "", "Lim1> [V]", "4.095", "", "", "", ""], ["", "", "", "", "", "", "", "", "", "", "", "", "", "", "", "", "", "", "", "", "", "", "", "", "", "", "", "", "Lim1< [uA]", "-40000", "", "", "", "", "", "", "", "", "", "", "", "", "Lim< [V]", "-4.095", "", "", "", ""], ["", "", "", "", "", "", "", "", "", "", "", "", "", "", "", "", "", "", "", "", "", "", "", "", "", "", "", "", "", "", "", "", "", "", "", "", "", "", "", "", "", "", "", "", "", "", "", ""], ["", "", "", "", "", "", "", "", "", "", "", "", "", "", "", "", "", "", "", "", "", "", "", "", "", "", "", "", "", "", "", "", "", "", "", "", "", "", "", "", "", "", "", "", "", "", "", ""], ["", "", "", "", "", "", "", "", "", "", "", "", "", "", "", "", "", "", "", "", "", "", "", "", "", "", "", "", "", "", "", "", "", "", "", "", "", "", "", "", "", "", "", "", "", "", "", ""], ["", "", "", "", "", "", "", "", "", "", "", "", "", "", "", "", "", "", "", "", "", "", "", "", "", "", "", "", "", "", "", "", "", "", "", "", "", "", "", "", "", "", "", "", "", "", "", ""], ["", "", "", "", "", "", "", "", "", "", "", "", "", "", "", "", "", "", "", "", "", "", "", "", "", "", "", "", "", "", "", "", "", "", "", "", "", "", "", "", "", "", "", "", "", "", "", ""]]  # Individual Pram
    w59 = string[][] [["LSV", "LSV", "CV", "CV", "SWV", "SWV", "DPV", "DPV", "NPV", "NPV", "NDPV", "NDPV", "ACV", "ACV", "LPR", "LPR", "LSV+AD", "LSV+AD", "CV+AD", "CV+AD", "AD", "AD", "ZRA", "ZRA", "FA", "FA", "PAD", "PAD", "MAD", "MAD", "COUL", "COUL", "LSP", "LSP", "CVP", "CVP", "POT", "POT", "ZCP", "ZCP", "FP", "FP", "MPD", "MPD", "PSAF", "PSAF", "PSAG", "PSAG"], ["3", "3", "3", "3", "4", "4", "5", "5", "5", "5", "7", "7", "6", "6", "6", "6", "6", "6", "7", "7", "2", "2", "2", "2", "2", "2", "12", "12", "2", "2", "2", "2", "3", "3", "3", "3", "2", "2", "2", "2", "2", "2", "2", "2", "2", "2", "3", "3"], ["Estep [V]", "0.002", "Estep [V]", "0.002", "Estep [V]", "0.005", "Estep [V]", "0.004 [V]", "Estep [V]", "0.005", "Estep [V]", "0.005 [V]", "Estep [V]", "0.008", "dE/dt lim [uV/s]", "1", "Ebegin [V]", "0.1", "Ebegin [V]", "0.1", "Interval [s]", "0.1", "Interval [s]", "0.5", "Interval [ms]", "50", "E1 [V]", "0.4", "Interval [s]", "0.1", "Interval [s]", "0.5", "Istep [uA]", "0.005", "Istep [uA]", "0.01", "Interval [s]", "0.5", "Interval [s]", "0.5", "Interval [ms]", "10", "Internal [s]", "0.1", "Elimit [V]", "1", "Elimit [V]", "1"], ["Srate [V/s]", "0.05", "Srate [V/s]", "0.05", "Eamp [V]", "0.002", "Epuls [V]", "0.002", "Ebase [V]", "0", "tint [ms]", "50", "Eamp [V]", "0.1", "tmaxOCP [s]", "120", "Eend [V]", "0.9", "Evtx1 [V]", "0.9", "t [s]", "3600", "t [s]", "20", "t [s]", "20", "t1 [s]", "0.1", "Repeat [times]", "1", "t[s]", "30", "Srate [uA/s]", "0.2", "Srate [uA/s]", "0.1", "t [s]", "60", "t [s]", "60", "t [s]", "5", "Repeat [times]", "1", "tmax [s]", "10", "S.Cur [uA]", "10"], ["nscans", "1", "nscans", "1", "Freq [Hz]", "20", "tpuls [ms]", "10", "tmod [ms]", "25", "Ebase [V]", "0", "tmod [ms]", "160", "tprecond [s]", "5", "E2 [V]", "1", "Evtx2 [V]", "-0.1", "", "", "", "", "", "", "E2 [V]", "-0.2", "", "", "", "", "Nscans", "1", "Nscans", "1", "", "", "", "", "", "", "", "", "", "", "tmax [s]", "10"], ["", "", "", "", "nscans", "1", "Srate [V/s]", "0.04", "tint [ms]", "100", "Epuls [V]", "0.003", "Freq [Hz]", "50", "Estep [V]", "0.001", "Estep [V]", "0.002", "E2 [V]", "0.1", "", "", "", "", "", "", "t2 [s]", "0.2", "", "", "", "", "", "", "", "", "", "", "", "", "", "", "", "", "", "", "", ""], ["", "", "", "", "", "", "nscans", "1", "nscans", "1", "tpuls [ms]", "10", "tint [ms]", "560 [ms]", "Srate [V/s]", "0.001", "Srate [V/s]", "0.05", "Estep [V]", "0.002", "", "", "", "", "", "", "E3 [V]", "0.41", "", "", "", "", "", "", "", "", "", "", "", "", "", "", "", "", "", "", "", ""], ["", "", "", "", "", "", "", "", "", "", "tmod [ms]", "10", "nscans", "1", "nscans", "1", "nscans", "1", "Srate [V/s]", "0.05", "", "", "", "", "", "", "t3 [s]", "0.1", "", "", "", "", "", "", "", "", "", "", "", "", "", "", "", "", "", "", "", ""], ["", "", "", "", "", "", "", "", "", "", "nscans", "1", "", "", "", "", "", "", "nscans", "1", "", "", "", "", "", "", "E4 [V]", "-0.2", "", "", "", "", "", "", "", "", "", "", "", "", "", "", "", "", "", "", "", ""], ["", "", "", "", "", "", "", "", "", "", "", "", "", "", "", "", "", "", "", "", "", "", "", "", "", "", "t4 [s]", "0.2", "", "", "", "", "", "", "", "", "", "", "", "", "", "", "", "", "", "", "", ""], ["", "", "", "", "", "", "", "", "", "", "", "", "", "", "", "", "", "", "", "", "", "", "", "", "", "", "E5 [V]", "0.4", "", "", "", "", "", "", "", "", "", "", "", "", "", "", "", "", "", "", "", ""], ["", "", "", "", "", "", "", "", "", "", "", "", "", "", "", "", "", "", "", "", "", "", "", "", "", "", "t5 [s]", "0.1", "", "", "", "", "", "", "", "", "", "", "", "", "", "", "", "", "", "", "", ""], ["", "", "", "", "", "", "", "", "", "", "", "", "", "", "", "", "", "", "", "", "", "", "", "", "", "", "ti [s]", "0.3", "", "", "", "", "", "", "", "", "", "", "", "", "", "", "", "", "", "", "", ""], ["", "", "", "", "", "", "", "", "", "", "", "", "", "", "", "", "", "", "", "", "", "", "", "", "", "", "t [s]", "20", "", "", "", "", "", "", "", "", "", "", "", "", "", "", "", "", "", "", "", ""]]  # Common Pram
    n29 = event shown="[2] \"Stop all\": Value Change" {
      selector: _ -> [_ _ _]
      dyn-events: _ -> [_ _ _]
      timeout: _ -> [_ _ _]
      tunnel: [_ "VISA resource name" _] -> w52
      tunnel: [_ "Serial Settings" _] -> w51
      tunnel: [_ _ TRUE] -> w49
      event Timeout {
        n30 = event-data() -> ()  [unwired: 1 in, 3 out]
      }
      event "Check port": Value Change {
        n31 = event-data() -> ()  [unwired: 1 in, 1 out]
      }
      event "Stop all": Value Change {
        n32 = event-data() -> ()  [unwired: 1 in, 1 out]
      }
    }
    n33 = control-ref of="Technique N 1"() -> (w85:refnum<vi>)
    n34 = control-ref of="Technique N 2"() -> (w84:refnum<vi>)
    n35 = control-ref of="Technique N 3"() -> (w83:refnum<vi>)
    n36 = control-ref of="Technique N 4"() -> (w82:refnum<vi>)
    n37 = control-ref of="Technique N 5"() -> (w81:refnum<vi>)
    n38 = control-ref of="Technique N 6"() -> (w80:refnum<vi>)
    n39 = control-ref of="Technique N 7"() -> (w79:refnum<vi>)
    n40 = control-ref of="Technique N 8"() -> (w78:refnum<vi>)
    n41 = control-ref of="Technique M"() -> (w77:refnum<vi>)
    n42 = Array Size(array=w58) -> (size(s)=w60:i32[])
    n43 = Array Size(array=w59) -> (size(s)=w68:i32[])
    n44 = Index Array(array=w60) -> (element #2=w61:i32)  [unwired: 2 in, 1 out]
    n45 = Index Array(array=w68) -> (element #2=w69:i32)  [unwired: 2 in, 1 out]
    n46 = control-ref of="Pretr N 1"() -> (w109:refnum<vi>)
    n47 = control-ref of="Pretr N 2"() -> (w108:refnum<vi>)
    n48 = control-ref of="Pretr N 3"() -> (w107:refnum<vi>)
    n49 = control-ref of="Pretr N 4"() -> (w106:refnum<vi>)
    n50 = control-ref of="Pretr N 5"() -> (w105:refnum<vi>)
    n51 = control-ref of="Pretr N 6"() -> (w104:refnum<vi>)
    n52 = control-ref of="Pretr N 7"() -> (w103:refnum<vi>)
    n53 = control-ref of="Pretr N 8"() -> (w102:refnum<vi>)
    n54 = control-ref of="Pretr M"() -> (w101:refnum<vi>)
    n55 = Build Array(w85, w84, w83, w82, w81, w80, w79, w78, w77) -> (w158:refnum<vi>[])
    n56 = Divide(x=w61, y=2) -> (x/y=w63:dbl)
    n57 = Divide(x=w69, y=2) -> (x/y=w71:dbl)
    n58 = call "Init.vi"("error in"=errorcluster {"status"=FALSE, "code"=0, "source"=""}, "Serial Settings"=w51, "VISA Refnum in"=w52) -> ("error out"=w54:errorcluster, "Device model"=w55:string, "Cluster"=w56:T12)  [unwired: 6 in]
    n59 = for {
      N: w63 -> [_]
      tunnel: w58 -> [w180]
      tunnel: [w176] -> w64 mode=indexing
      tunnel: [w175] -> w65 mode=indexing
      i -> [w179]
      n60 = Multiply(x=w179, y=2) -> (x*y=w178:i32)
      n61 = Index Array(array=w180, index (col) #1=w178) -> (element #1=w176:string[], element #2=w175:string[])  [unwired: 3 in]
    }
    n62 = for {
      N: w71 -> [_]
      tunnel: w59 -> [w186]
      tunnel: [w182] -> w72 mode=indexing
      tunnel: [w181] -> w73 mode=indexing
      i -> [w185]
      n63 = Multiply(x=w185, y=2) -> (x*y=w184:i32)
      n64 = Index Array(array=w186, index (col) #1=w184) -> (element #1=w182:string[], element #2=w181:string[])  [unwired: 3 in]
    }
    n65 = Build Array(w109, w108, w107, w106, w105, w104, w103, w102, w101) -> (w156:refnum<vi>[])
    n66 = Build Array(string[][] [["Econd [V]", "Icond [uA]"], ["Tcond [s]", "Tcond [s]"], ["Edep [V]", "Idep [uA]"], ["Tdep [s]", "Tdep [s]"], ["Tequil [s]", "Tequil [s]"]], string[][] [["0", "0", "0"], ["0", "0", "0"], ["0", "0", "0"], ["0", "0", "1"], ["3", "0", "0"]]) -> (w110:string[][][])
    n67 = control-ref of="Parameters N 1"() -> (w87:refnum<vi>)
    n68 = control-ref of="Parameters N 2"() -> (w88:refnum<vi>)
    n69 = control-ref of="Parameters N 3"() -> (w89:refnum<vi>)
    n70 = control-ref of="Parameters N 4"() -> (w90:refnum<vi>)
    n71 = control-ref of="Parameters N 5"() -> (w91:refnum<vi>)
    n72 = control-ref of="Parameters N 6"() -> (w92:refnum<vi>)
    n73 = control-ref of="Parameters N 7"() -> (w86:refnum<vi>)
    n74 = control-ref of="Parameters N 8"() -> (w93:refnum<vi>)
    n75 = control-ref of="Parameters M"() -> (w94:refnum<vi>)
    n76 = control-ref of="Node list"() -> (w98:refnum<vi>)
    n77 = Bundle(w156, w110) -> (w155:cluster{refnum<vi>[], string[][][]})  [unwired: 1 in]
    n78 = Transpose 2D Array(2D array=w64) -> (transposed array=w66:string[][])
    n79 = Transpose 2D Array(2D array=w65) -> (transposed array=w67:string[][])
    n80 = Transpose 2D Array(2D array=w72) -> (transposed array=w74:string[][])
    n81 = Transpose 2D Array(2D array=w73) -> (transposed array=w75:string[][])
    n82 = Build Array(w87, w88, w89, w90, w91, w92, w86, w93, w94) -> (w157:refnum<vi>[])
    n83 = Build Array(w66, w67) -> (w153:string[][][])
    n84 = Build Array(w74, w75) -> (w154:string[][][])
    n85 = call "Tree Init.vi"("Model"=w55, "TreeControl in"=w98) -> ("error out"=w100:errorcluster, "TreeControl out"=w99:refnum<vi>)  [unwired: 8 in]
    n86 = property class="Tree (strict)"(reference=w99, error in=w100, "Value"=string[] ["Node 1 - Ch1"]) -> (reference out=w76:refnum<vi>)  [unwired: 1 out]
    n87 = Bundle By Name(cluster=w56, "Tree 2"=w76) -> (w96:T12)
    n88 = call "Param Controls Updates.vi"("Individual Pram"=w153, "Pretreatment"=w155, "Common Pram"=w154, "Accept St"=TRUE, "error in (no error)"=w54, "Technique"=w158, "Parameters"=w157, "Reference in"=w96) -> ("error out"=w160:errorcluster, "Reference out"=w159:T12)  [unwired: 2 in]
    n89 = case shown="Error .." w160 {
      tunnel: [FALSE TRUE] -> w57
      frame No Error {
      }
      frame Error {
      }
    }
    n90 = Not(x=w57) -> (.not. x?=w50:bool)
    n91 = local write "Status"(w57) -> ()
    n92 = Or(x=w50, y=w49) -> (x .or. y?=w48:bool)
    "potentiostat" <- w48
    n93 = case shown="False" w48 {
      selector: w48 -> [_ w167]
      tunnel: w160 -> [w166 w169]
      tunnel: w159 -> [w165 w168]
      tunnel: [w164 w169] -> w152
      tunnel: [w163 w168] -> w149
      tunnel: [w162 w167] -> w115
      frame False {
        n94 = call "Technique Selection 2.vi"("error in (no error)"=w166, "Reference In"=w165) -> ("error out"=w164:errorcluster, "Accept St"=w162:bool, "Reference Out"=w163:T12)  [unwired: 5 in, 2 out]
      }
      frame True {
      }
    }
    n95 = call "Param Controls Updates.vi"("Individual Pram"=w153, "Pretreatment"=w155, "Common Pram"=w154, "Accept St"=w115, "error in (no error)"=w152, "Technique"=w158, "Parameters"=w157, "Reference in"=w149) -> ("error out"=w151:errorcluster, "Reference out"=w148:T12)  [unwired: 2 in]
    n96 = control-ref of="Option N 1"() -> (w146:refnum<vi>)
    n97 = control-ref of="Option N 2"() -> (w145:refnum<vi>)
    n98 = control-ref of="Option N 3"() -> (w144:refnum<vi>)
    n99 = control-ref of="Option N 4"() -> (w143:refnum<vi>)
    n100 = control-ref of="Option N 5"() -> (w142:refnum<vi>)
    n101 = control-ref of="Option N 6"() -> (w141:refnum<vi>)
    n102 = control-ref of="Option N 7"() -> (w140:refnum<vi>)
    n103 = control-ref of="Option N 8"() -> (w139:refnum<vi>)
    n104 = control-ref of="Option M"() -> (w138:refnum<vi>)
    n105 = control-ref of="CR N 1"() -> (w137:refnum<vi>)
    n106 = control-ref of="CR N 2"() -> (w136:refnum<vi>)
    n107 = control-ref of="CR N 3"() -> (w135:refnum<vi>)
    n108 = control-ref of="CR N 4"() -> (w134:refnum<vi>)
    n109 = control-ref of="CR N 5"() -> (w133:refnum<vi>)
    n110 = control-ref of="CR N 6"() -> (w132:refnum<vi>)
    n111 = control-ref of="CR N 7"() -> (w131:refnum<vi>)
    n112 = control-ref of="CR N 8"() -> (w130:refnum<vi>)
    n113 = Build Array(w137, w136, w135, w134, w133, w132, w131, w130) -> (w128:refnum<vi>[])
    n114 = Build Array(w146, w145, w144, w143, w142, w141, w140, w139, w138) -> (w129:refnum<vi>[])
    n115 = control-ref of="Config Status"() -> (w119:refnum<vi>)
    n116 = call "Command List 400.vi"("Byte count"=2000, "Parameters"=w157, "Status"=w119, "Pretreatment"=w156, "error in (no error)"=w151, "CR"=w128, "Options"=w129, "Reference in"=w148) -> ("error out"=w150:errorcluster, "Interval"=w123:dbl[], "St Cell"=w121:bool, "Reference out"=w147:T12)
    n117 = Array Max & Min(array=w123) -> (max value=w126:dbl)  [unwired: 3 out]
    n118 = call "Start Task.vi"("Timeout"=w126, "error in (no error)"=w150, "Reference In"=w147) -> ("error out"=w124:errorcluster, "Reference Out"=w125:T12)  [unwired: 6 in, 1 out]
    n119 = while {
      tunnel: w125 -> [w202]
      tunnel: w124 -> [w201]
      stop <- w199 stop-if-true
      n120 = control-ref of="result"() -> (w200:refnum<vi>)
      n121 = call "Data Read.vi"("error in (no error)"=w201, "result 2"=w200, "Reference In"=w202) -> ("error out"=w197:errorcluster)  [unwired: 7 in, 1 out]
      n122 = local read "result"() -> (w198:bool)
      n123 = Or(x=w198, y=w197) -> (x .or. y?=w199:bool)
    }
    n124 = while {
      tunnel: w125 -> [w215]
      tunnel: w123 -> [w214]
      tunnel: w124 -> [w213]
      tunnel: [w212] -> w120
      tunnel: [w211] -> w114
      tunnel: ["stop Measuring"] -> w118
      i -> [w204]
      stop <- w206 stop-if-true
      n125 = Equal To 0?(x=w204) -> (x = 0?=w203:bool)
      n126 = call "Data analysis.vi"("First Call"=w203, "error in (no error)"=w213, "Interval"=w214, "Reference In"=w215) -> ("error out"=w211:errorcluster, "Actual Values"=w209:T10, "Reference Out"=w212:T12, "Stop"=w208:bool, "Array 2"=→"Curves":cluster{dbl[], dbl[]}[])  [unwired: 3 in]
      "Actual Values" <- w209
      "result" <- w208
      n127 = Compound Arithmetic op=OR(w211, w208, "stop Measuring") -> (w206:bool)
      n128 = Unbundle(w209) -> ("Actual I/U"=→"Actual I/U 2":dbl)  [unwired: 2 out]
    }
    n129 = case shown="Error" w114 {
      selector: w114 -> [w187 w189]
      tunnel: [w187 w188] -> w113
      frame No Error {
      }
      frame Error {
        n130 = Unbundle By Name "Unbundle By Name"(w189) -> ("code"=w192:i32)
        n131 = Equal?(x=w192, y=-1073807339) -> (x = y?=w190:bool)
        n132 = case shown="True" w190 {
          tunnel: w189 -> [w193 w196]
          tunnel: [w193 w194] -> w188
          frame False {
          }
          frame True {
            n133 = Bundle By Name(cluster=w196, "status"=FALSE) -> (w194:errorcluster)
          }
        }
      }
    }
    n134 = call "Stop Task.vi"("error in (no error)"=w113, "Stop meas"=w118, "St Cell"=w121, "Reference In"=w120) -> ("error out"=w116:errorcluster, "Reference Out"=w117:T12)  [unwired: 6 in]
    "error out" <- w116
    n135 = Unbundle By Name(w116) -> ("status"=→"Status":bool)
    n136 = call "Close.vi"("error in (no error)"=w116, "Reference Out"=w117) -> ()  [unwired: 9 in, 1 out]
    "Status" <- FALSE ("Status")
  }
  n137 = local write "Sent value"(w32) -> ()
  n138 = while {
    tunnel: w3 -> [w218]
    stop <- w216 stop-if-true
    n139 = local read "Stop all"() -> (w216:bool)
    "Camera" <- w216
    n140 = call "Vision Acquisition"("Stop (F)"=w216) -> ("Image Out"=→"Image Out":T8)  [unwired: 24 in, 2 out]
    n141 = Not(x=w216) -> (.not. x?=w217:bool)
    n142 = case shown="False" w217 {
      selector: w217 -> [w220 _]
      tunnel: w218 -> [w224 _]
      frame False {
        n143 = flat-sequence {
          tunnel: w220 -> [w228]
          tunnel: ["set abort"] -> w226
          tunnel: ["\r\n"] -> w227
          frame #0 {
            n144 = local write "XYXA"(w228) -> ()
            n145 = local write "manual"(w228) -> ()
            n146 = Wait (ms)(milliseconds to wait=u32 101) -> ()  [unwired: 1 out]
          }
          frame #1 {
          }
        }
        n147 = Concatenate Strings(w226, w227) -> (w225:string)
        n148 = TCP Write(connection ID=w224, data in=w225) -> (connection ID out=w223:refnum<k5>, bytes written=w222:i32)  [unwired: 2 in, 1 out]
        n149 = call "set_read.vi"("connection ID"=w223, "bytes to read"=w222) -> ("concatenated string"=w221:string)  [unwired: 4 in, 1 out]
        n150 = local write "MDI"(w221) -> ()
      }
      frame True {
      }
    }
  }
  n151 = while {
    tunnel: w3 -> [w236]
    tunnel: string[] ["X", "Y", "Z", "A"] -> [w241]
    tunnel: string[] [] -> [w239]
    tunnel: string[][] [] -> [w238]
    tunnel: string[] ["X ", "X -", "Y ", "Y -", "Z ", "Z -", "A ", "A -"] -> [w237]
    shift-right: [w234] -> _
    shift-left: T11."Enable all" ("Enum") -> [w235]
    shift-right: [w232] -> _
    shift-left: dbl[] [0.0, 0.0, 0.0, 0.0] -> [w233]
    stop <- w240 stop-if-true
    n152 = case shown="\"Move to target\"" w235 {
      tunnel: w236 -> [_ w442 w548 _ _ _]
      tunnel: w241 -> [w249 _ _ _ _ _]
      tunnel: [w248 FALSE ("NewVal") FALSE ("NewVal") FALSE ("NewVal") w695 _] -> w240
      tunnel: w239 -> [w247 _ _ _ _ _]
      tunnel: w238 -> [w246 _ _ _ _ _]
      tunnel: w237 -> [w245 _ _ _ _ _]
      tunnel: w236 -> [w244 _ _ _ _ _]
      tunnel: [w243 T11."Enable all" ("Enum") T11."Enable all" ("Enum") T11."Main" ("Enum") T11."Enable all" ("Enum") T11."Enable all" ("Enum")] -> w234
      tunnel: w233 -> [_ _ _ _ w694 _]
      tunnel: [w242 _ _ _ _ _] -> w232
      frame "Main", Default {
        n153 = event shown="[8] \"Area start\": Value Change" {
          selector: _ -> [_ _ _ _ _ _ _ _ _]
          dyn-events: _ -> [_ _ _ _ _ _ _ _ _]
          timeout: _ -> [_ _ _ _ _ _ _ _ _]
          tunnel: w246 -> [_ _ _ _ _ _ _ _ _]
          tunnel: [_ w251 _ _ _ _ _ _ _] -> w248
          tunnel: w244 -> [_ _ _ w261 w280 w305 _ _ _]
          tunnel: w249 -> [_ _ _ _ w279 _ _ _ _]
          tunnel: w245 -> [_ _ _ _ _ w308 _ _ _]
          tunnel: [T11."Enable all" ("Enum") _ _ T11."Move to target" ("Enum") T11."Move to target" ("Enum") w304 _ T11."Line" ("Enum") T11."Area Move" ("Enum")] -> w243
          tunnel: [_ _ _ dbl[] [0.5, 0.5, 0.5, 0.0] w272 w303 _ _ _] -> w242
          event Timeout {
            n154 = event-data() -> ()  [unwired: 1 in, 1 out]
          }
          event "Stop all": Value Change {
            n155 = event-data() -> ("NewVal"=w251:bool)  [unwired: 1 in]
          }
          event "Copy current position": Value Change {
            n156 = event-data() -> ()  [unwired: 1 in, 1 out]
            n157 = local read "True A"() -> (w255:dbl)
            n158 = local read "True Z"() -> (w254:dbl)
            n159 = local read "True Y"() -> (w253:dbl)
            n160 = local read "True X"() -> (w252:dbl)
            n161 = local write "A"(w255) -> ()
            n162 = local write "Z"(w254) -> ()
            n163 = local write "Y"(w253) -> ()
            n164 = local write "X"(w252) -> ()
          }
          event "Home": Value Change {
            n165 = event-data() -> ()  [unwired: 1 in, 1 out]
            n166 = Concatenate Strings("set home 0 ", "\r\n", "set home 1 ", "\r\n", "set home 2 ", "\r\n", "set home 3 ", "\r\n") -> (w270:string)
            n167 = TCP Write(connection ID=w261, data in=w270) -> (connection ID out=w258:refnum<k5>, bytes written=w259:i32)  [unwired: 2 in, 1 out]
            n168 = call "set_read.vi"("connection ID"=w258, "bytes to read"=w259) -> ("concatenated string"=w260:string)  [unwired: 4 in, 1 out]
            n169 = local write "MDI"(w260) -> ()
          }
          event "Move": Value Change {
            n170 = event-data() -> ()  [unwired: 1 in, 1 out]
            n171 = Build Array("X", "Y", "Z", "A") -> (w272:dbl[])
            n172 = for {
              tunnel: w279 -> [w296] mode=indexing
              tunnel: w272 -> [w297] mode=indexing
              tunnel: [w294] -> w278 mode=indexing
              i -> [w293]
              n173 = Equal?(x=w293, y=3) -> (x = y?=w291:bool)
              n174 = Format Into String(format string="%#f", w297) -> (resulting string=w295:string)  [unwired: 2 in, 1 out]
              n175 = call <vilib>:"Space Constant.vi"() -> ("String"=w290:string)
              n176 = Select(t="", s=w291, f=w290) -> (s? t:f=w289:string)
              n177 = Concatenate Strings(w296, w295, w289) -> (w294:string)
            }
            n178 = Array To Spreadsheet String(array=w278, 3:"%s" ("format string")) -> (spreadsheet string=w277:string)  [unwired: 1 in]
            n179 = Concatenate Strings("set mdi G0 ", w277, "\r\n") -> (w275:string)
            "Sent value" <- w275
            n180 = TCP Write(connection ID=w280, data in=w275) -> (connection ID out=w281:refnum<k5>, bytes written=w282:i32)  [unwired: 2 in, 1 out]
            n181 = call "set_read.vi"("connection ID"=w281, "bytes to read"=w282) -> ("concatenated string"=w283:string)  [unwired: 4 in, 1 out]
            n182 = local write "MDI"(w283) -> ()
          }
          event "x+", "x-", "y+", "y-", "z+", "z-": Value Change {
            n183 = event-data() -> ()  [unwired: 1 in, 1 out]
            n184 = Build Array("x+", "x-", "y+", "y-", "z+", "z-", "A+", "A-") -> (w311:bool[])
            n185 = Search 1D Array(1D array=w311, element=TRUE) -> (index of element=w307:i32)  [unwired: 1 in]
            n186 = local read "Jog?"() -> (w306:bool)
            n187 = Less Than 0?(x=w307) -> (x < 0?=w309:bool)
            n188 = case shown="True" w306 {
              tunnel: w309 -> [w321 w385]
              tunnel: w308 -> [w319 w383]
              tunnel: w307 -> [w320 w380]
              tunnel: w305 -> [w318 w382]
              tunnel: [w317 w381] -> w304
              tunnel: [w316 _] -> w303
              frame False {
                n189 = case shown="False" w321 {
                  tunnel: w320 -> [w322 _]
                  tunnel: w319 -> [w350 _]
                  tunnel: w318 -> [w339 _]
                  tunnel: [T11."Move to target" ("Enum") T11."Move to target" ("Enum")] -> w317
                  tunnel: [w338 _] -> w316
                  frame False {
                    n190 = Index Array(array=w350, index=w322) -> (element=w329:string)
                    n191 = Quotient & Remainder(x=w322, y=2) -> (floor(x/y)=w324:i32)  [unwired: 1 out]
                    n192 = case shown="\"X \", Default" w329 {
                      tunnel: "Step size (mm)" -> [w353 w356 w360 w364 w368 w372]
                      tunnel: [w352 w358 w362 w366 w370 w374] -> w328
                      tunnel: ["X" "X" "Y" "Y" "Z" "Z"] -> w325
                      frame "X ", Default {
                        n193 = local read "True X"() -> (w354:dbl)
                        n194 = Add(x=w354, y=w353) -> (x+y=w352:dbl)
                      }
                      frame "X -" {
                        n195 = local read "True X"() -> (w357:dbl)
                        n196 = Subtract(x=w357, y=w356) -> (x-y=w358:dbl)
                      }
                      frame "Y " {
                        n197 = local read "True Y"() -> (w361:dbl)
                        n198 = Add(x=w361, y=w360) -> (x+y=w362:dbl)
                      }
                      frame "Y -" {
                        n199 = local read "True Y"() -> (w365:dbl)
                        n200 = Subtract(x=w365, y=w364) -> (x-y=w366:dbl)
                      }
                      frame "Z " {
                        n201 = local read "True Z"() -> (w369:dbl)
                        n202 = Add(x=w369, y=w368) -> (x+y=w370:dbl)
                      }
                      frame "Z -" {
                        n203 = local read "True Z"() -> (w373:dbl)
                        n204 = Subtract(x=w373, y=w372) -> (x-y=w374:dbl)
                      }
                    }
                    n205 = Format Into String(format string="%#f", w328) -> (resulting string=w327:string)  [unwired: 2 in, 1 out]
                    n206 = TCP Write(connection ID=w339, data in="set mode mdi\n") -> (connection ID out=w344:refnum<k5>, bytes written=w343:i32)  [unwired: 2 in, 1 out]
                    n207 = Concatenate Strings("set mdi G0", w325, w327, "\r\n") -> (w346:string)
                    n208 = call "set_read.vi"("connection ID"=w344, "bytes to read"=w343) -> ("connection ID 2"=w342:refnum<k5>, "concatenated string"=w340:string)  [unwired: 4 in]
                    n209 = local read "True A"() -> (w337:dbl)
                    n210 = local read "True X"() -> (w335:dbl)
                    n211 = local read "True Y"() -> (w334:dbl)
                    n212 = local read "True Z"() -> (w336:dbl)
                    n213 = local write "MDI"(w340) -> ()
                    n214 = TCP Write(connection ID=w342, data in=w346) -> (connection ID out=w349:refnum<k5>, bytes written=w348:i32)  [unwired: 2 in, 1 out]
                    n215 = call "set_read.vi"("connection ID"=w349, "bytes to read"=w348) -> ("concatenated string"=w345:string)  [unwired: 4 in, 1 out]
                    n216 = Build Array(w335, w334, w336, w337) -> (w333:dbl[])
                    n217 = flat-sequence {
                      tunnel: w345 -> [w375]
                      frame #0 {
                        n218 = local write "MDI"(w375) -> ()
                      }
                      frame #1 {
                        n219 = local write "XYXA"(TRUE ("XYXA")) -> ()
                      }
                    }
                    n220 = Replace Array Subset(array=w333, new element=w328, index=w324) -> (w338:dbl[])
                  }
                  frame True {
                  }
                }
              }
              frame True {
                n221 = Quotient & Remainder(x=w380, y=2) -> (floor(x/y)=→"Moving":i32)  [unwired: 1 out]
                n222 = Multiply(x="Speed (mm/s) manual", y=1.0) -> (x*y=w389:dbl)
                n223 = Format Into String(format string="%#f", w389) -> (resulting string=w384:string)  [unwired: 2 in, 1 out]
                n224 = case shown="False" w385 {
                  tunnel: w384 -> [w392 _]
                  tunnel: w383 -> [w408 _]
                  tunnel: w380 -> [w407 _]
                  tunnel: w382 -> [w391 w415]
                  tunnel: [T11."Main" ("Enum") w412] -> w381
                  frame False {
                    n225 = Index Array(array=w408, index=w407) -> (element=w393:string)
                    n226 = Concatenate Strings("set mode manual", "\r\n") -> (w397:string)
                    n227 = TCP Write(connection ID=w391, data in=w397) -> (connection ID out=w406:refnum<k5>, bytes written=w405:i32)  [unwired: 2 in, 1 out]
                    n228 = call "set_read.vi"("connection ID"=w406, "bytes to read"=w405) -> ("connection ID 2"=w401:refnum<k5>, "concatenated string"=w404:string)  [unwired: 4 in]
                    n229 = Concatenate Strings("set jog ", w393, w392, "\r\n") -> (w400:string)
                    n230 = local write "MDI"(w404) -> ()
                    n231 = TCP Write(connection ID=w401, data in=w400) -> (connection ID out=w403:refnum<k5>, bytes written=w402:i32)  [unwired: 2 in, 1 out]
                    n232 = call "set_read.vi"("connection ID"=w403, "bytes to read"=w402) -> ("concatenated string"=w399:string)  [unwired: 4 in, 1 out]
                    n233 = flat-sequence {
                      tunnel: w399 -> [w410]
                      frame #0 {
                        n234 = local write "MDI"(w410) -> ()
                        n235 = Wait (ms)(milliseconds to wait=u32 101) -> ()  [unwired: 1 out]
                      }
                      frame #1 {
                        n236 = local write "manual"(TRUE ("manual")) -> ()
                      }
                    }
                  }
                  frame True {
                    n237 = flat-sequence {
                      tunnel: ["\r\n"] -> w414
                      frame #0 {
                        n238 = local write "manual"(FALSE ("manual")) -> ()
                        n239 = Wait (ms)(milliseconds to wait=u32 51) -> ()  [unwired: 1 out]
                      }
                      frame #1 {
                      }
                    }
                    n240 = Concatenate Strings("set abort", w414) -> (w421:string)
                    n241 = TCP Write(connection ID=w415, data in=w421) -> (connection ID out=w423:refnum<k5>, bytes written=w424:i32)  [unwired: 2 in, 1 out]
                    n242 = call "set_read.vi"("connection ID"=w423, "bytes to read"=w424) -> ("connection ID 2"=w413:refnum<k5>, "concatenated string"=w422:string)  [unwired: 4 in]
                    n243 = local write "MDI"(w422) -> ()
                    n244 = Concatenate Strings("set mode mdi", "\r\n") -> (w420:string)
                    n245 = TCP Write(connection ID=w413, data in=w420) -> (connection ID out=w425:refnum<k5>, bytes written=w426:i32)  [unwired: 2 in, 1 out]
                    n246 = call "set_read.vi"("connection ID"=w425, "bytes to read"=w426) -> ("concatenated string"=w419:string)  [unwired: 4 in, 1 out]
                    n247 = flat-sequence {
                      tunnel: w419 -> [w428]
                      tunnel: [T11."Enable all" ("Enum")] -> w412
                      frame #0 {
                        n248 = local write "MDI"(w428) -> ()
                        n249 = Wait (ms)(milliseconds to wait=u32 30) -> ()  [unwired: 1 out]
                      }
                      frame #1 {
                      }
                    }
                  }
                }
              }
            }
          }
          event "Jog?": Value Change {
            n250 = event-data() -> ()  [unwired: 1 in, 1 out]
            n251 = Not(x="Jog?") -> (.not. x?=w433:bool)
            "Step" <- w433
            n252 = property on="Step size (mm)" class="DigNum (strict)"("Visible"=w433) -> ()  [unwired: 2 in, 2 out]
            n253 = property on="Speed (mm/s) manual" class="Knob (strict)"("Visible"="Jog?") -> ()  [unwired: 2 in, 2 out]
            n254 = property on="stop step" class="Bool"("Visible"=w433) -> ()  [unwired: 2 in, 2 out]
            "Jog" <- "Jog?"
          }
          event "2D start": Value Change {
            w436 = T14."Disabled and Grayed Out" ("Disabled")
            n255 = event-data() -> ()  [unwired: 1 in, 1 out]
            n256 = property on="X0" class="DigNum (strict)"("DisabledEnum"=w436) -> ()  [unwired: 2 in, 2 out]
            n257 = property on="X1" class="DigNum (strict)"("DisabledEnum"=w436) -> ()  [unwired: 2 in, 2 out]
            n258 = property on="No. of teps" class="DigNum (strict)"("DisabledEnum"=w436) -> ()  [unwired: 2 in, 2 out]
            n259 = property on="Y0" class="DigNum (strict)"("DisabledEnum"=w436) -> ()  [unwired: 2 in, 2 out]
            n260 = property on="Y1" class="DigNum (strict)"("DisabledEnum"=w436) -> ()  [unwired: 2 in, 2 out]
            n261 = property on="Speed (micron/s) 2D" class="Knob (strict)"("DisabledEnum"=w436) -> ()  [unwired: 2 in, 2 out]
            n262 = property on="Wait (ms)" class="DigNum (strict)"("DisabledEnum"=w436) -> ()  [unwired: 2 in, 2 out]
          }
          event "Area start": Value Change {
            w438 = T14."Disabled and Grayed Out" ("Disabled")
            n263 = event-data() -> ()  [unwired: 1 in, 1 out]
            n264 = property on="x1" class="DigNum (strict)"("DisabledEnum"=w438) -> ()  [unwired: 2 in, 2 out]
            n265 = property on="y0" class="DigNum (strict)"("DisabledEnum"=w438) -> ()  [unwired: 2 in, 2 out]
            n266 = property on="Line displacement" class="DigNum (strict)"("DisabledEnum"=w438) -> ()  [unwired: 2 in, 2 out]
            n267 = property on="Speed (micron/s) A" class="Knob (strict)"("DisabledEnum"=w438) -> ()  [unwired: 2 in, 2 out]
            n268 = property on="y1" class="DigNum (strict)"("DisabledEnum"=w438) -> ()  [unwired: 2 in, 2 out]
            n269 = property on="Step size" class="DigNum (strict)"("DisabledEnum"=w438) -> ()  [unwired: 2 in, 2 out]
            n270 = property on="x0" class="DigNum (strict)"("DisabledEnum"=w438) -> ()  [unwired: 2 in, 2 out]
            n271 = property on="Wait (ms) Area" class="DigNum (strict)"("DisabledEnum"=w438) -> ()  [unwired: 2 in, 2 out]
          }
        }
        "ArAx" <- w247
        "ArAy" <- w247
      }
      frame "Line" {
        w439 = TRUE ("Visible")
        # "Make sure to put the minimum and maximum positions in the properties"
        n272 = property on="YV Graph" class="XYGraph (strict)"("Visible"=w439) -> ()  [unwired: 2 in, 2 out]
        n273 = property on="XI/YI" class="Bool (strict)"("Visible"=w439) -> ()  [unwired: 2 in, 2 out]
        n274 = Subtract(x="X1", y="X0") -> (x-y=w447:dbl)
        n275 = Subtract(x="Y1", y="Y0") -> (x-y=w448:dbl)
        n276 = Equal?(x="X0", y="X1") -> (x = y?=w458:bool)
        n277 = Equal?(x="Y0", y="Y1") -> (x = y?=w459:bool)
        n278 = Divide(x=w448, y="No. of teps") -> (x/y=w454:dbl)
        n279 = Divide(x=w447, y="No. of teps") -> (x/y=w443:dbl)
        n280 = And(x=w458, y=w459) -> (x .and. y?=w449:bool)
        n281 = Multiply(x="Speed (micron/s) 2D", y=0.06) -> (x*y=w457:dbl)
        n282 = Format Into String(format string="%#f", w457) -> (resulting string=w455:string)  [unwired: 2 in, 1 out]
        n283 = case shown="False" w449 {
          tunnel: "No. of teps" -> [w464 _]
          tunnel: w454 -> [w463 _]
          tunnel: w455 -> [w462 _]
          tunnel: w443 -> [w461 _]
          tunnel: w442 -> [w460 _]
          frame False {
            n284 = Increment(x=w464) -> (x+1=w465:dbl)
            n285 = for {
              N: w465 -> [_]
              tunnel: w463 -> [w494]
              tunnel: w462 -> [w485]
              tunnel: w461 -> [w492]
              tunnel: w460 -> [w484]
              shift-right: [w468] -> _
              shift-left: _ -> [w471]
              shift-right: [w467] -> _
              shift-left: _ -> [w470]
              shift-right: [w466] -> _
              shift-left: _ -> [w469]
              i -> [w498]
              stop <- w475 stop-if-true
              w478 = "%3.3f" ("format string")
              n286 = local read "Y0"() -> (w493:dbl)
              n287 = local read "X0"() -> (w495:dbl)
              n288 = Multiply(x=w492, y=w498) -> (x*y=w496:dbl)
              n289 = Multiply(x=w498, y=w494) -> (x*y=w497:dbl)
              n290 = Add(x=w495, y=w496) -> (x+y=w480:dbl)
              n291 = Add(x=w497, y=w493) -> (x+y=w479:dbl)
              n292 = Bundle("Xarray"=w471, "Iarray"=w469) -> (→"XV Graph":cluster{"Xarray":dbl[], "Iarray":dbl[]})  [unwired: 1 in]
              n293 = Bundle("Yarray"=w470, "Iarray"=w469) -> (→"YV Graph":cluster{"Yarray":dbl[], "Iarray":dbl[]})  [unwired: 1 in]
              n294 = Format Into String(format string="%#f", w480) -> (resulting string=w482:string)  [unwired: 2 in, 1 out]
              n295 = Format Into String(format string=w478, w479) -> (resulting string=w476:string)  [unwired: 2 in, 1 out]
              n296 = Format Into String(format string="%#f", w479) -> (resulting string=w481:string)  [unwired: 2 in, 1 out]
              n297 = Format Into String(format string=w478, w480) -> (resulting string=w477:string)  [unwired: 2 in, 1 out]
              n298 = Concatenate Strings("set mdi G1 X", w482, " Y" ("string"), w481, " F" ("string"), w485, "\r\n") -> (w483:string)
              n299 = flat-sequence {
                tunnel: w484 -> [w509]
                tunnel: w483 -> [w508]
                tunnel: [w506] -> w474
                tunnel: [w515] -> w475
                tunnel: w477 -> [w514]
                tunnel: w476 -> [w513]
                tunnel: [w543] -> w468
                tunnel: [w542] -> w467
                tunnel: [w541] -> w466
                frame #0 {
                  n300 = TCP Write(connection ID=w509, data in=w508) -> (connection ID out=w510:refnum<k5>, bytes written=w511:i32)  [unwired: 2 in, 1 out]
                  n301 = call "set_read.vi"("connection ID"=w510, "bytes to read"=w511) -> ("connection ID 2"=w506:refnum<k5>, "concatenated string"=w507:string)  [unwired: 4 in]
                  n302 = local write "MDI"(w507) -> ()
                }
                frame #1 {
                  n303 = local write "XYXA"(TRUE ("XYXA")) -> ()
                }
                frame #2 {
                  n304 = while {
                    tunnel: ["2D stop"] -> w515
                    tunnel: w514 -> [w520]
                    tunnel: w513 -> [w519]
                    stop <- w528 stop-if-true
                    n305 = local read "True X"() -> (w524:dbl)
                    n306 = local read "True Y"() -> (w522:dbl)
                    n307 = Format Into String(format string="%3.3f", w524) -> (resulting string=w523:string)  [unwired: 2 in, 1 out]
                    n308 = Format Into String(format string="%3.3f", w522) -> (resulting string=w521:string)  [unwired: 2 in, 1 out]
                    n309 = Equal?(x=w521, y=w519) -> (x = y?=w517:bool)
                    n310 = Equal?(x=w523, y=w520) -> (x = y?=w516:bool)
                    n311 = Wait (ms)(milliseconds to wait=u32 1) -> ()  [unwired: 1 out]
                    n312 = And(x=w516, y=w517) -> (x .and. y?=w518:bool)
                    n313 = Or(x=w518, y="2D stop") -> (x .or. y?=w528:bool)
                  }
                }
                frame #3 {
                  n314 = local write "XYXA"(FALSE ("XYXA")) -> ()
                  n315 = Wait (ms)(milliseconds to wait="Wait (ms)") -> ()  [unwired: 1 out]
                }
                frame #4 {
                  n316 = local read "Actual I/U 2"() -> (w533:dbl)
                  n317 = local read "Iarray"() -> (w534:dbl[])
                  n318 = local read "Yarray"() -> (w535:dbl[])
                  n319 = local read "Xarray"() -> (w536:dbl[])
                  n320 = local read "True Y"() -> (w538:dbl)
                  n321 = local read "True X"() -> (w539:dbl)
                  n322 = Build Array(w533) -> (w532:dbl[])
                  n323 = Build Array(w538) -> (w537:dbl[])
                  n324 = Build Array(w539) -> (w540:dbl[])
                  n325 = Insert Into Array(array=w536, new element=w540) -> (w543:dbl[])  [unwired: 1 in]
                  n326 = Insert Into Array(array=w535, new element=w537) -> (w542:dbl[])  [unwired: 1 in]
                  n327 = Insert Into Array(array=w534, new element=w532) -> (w541:dbl[])  [unwired: 1 in]
                  n328 = local write "Xarray"(w543) -> ()
                  n329 = local write "Yarray"(w542) -> ()
                  n330 = local write "Iarray"(w541) -> ()
                }
              }
              n331 = case shown="True" w475 {
                tunnel: w474 -> [_ w503]
                frame False {
                }
                frame True {
                  n332 = Concatenate Strings("set abort", "\r\n") -> (w502:string)
                  n333 = TCP Write(connection ID=w503, data in=w502) -> (connection ID out=w505:refnum<k5>, bytes written=w504:i32)  [unwired: 2 in, 1 out]
                  n334 = call "set_read.vi"("connection ID"=w505, "bytes to read"=w504) -> ("concatenated string"=w499:string)  [unwired: 4 in, 1 out]
                  n335 = local write "MDI"(w499) -> ()
                }
              }
            }
          }
          frame True {
          }
        }
      }
      frame "Area Move" {
        n336 = Equal?(x="x0", y="x1") -> (x = y?=w566:bool)
        n337 = Subtract(x="x1", y="x0") -> (x-y=w569:dbl)
        n338 = Subtract(x="y1", y="y0") -> (x-y=w567:dbl)
        n339 = Equal?(x="y0", y="y1") -> (x = y?=w554:bool)
        n340 = Less?(x=w569, y="Step size") -> (x < y?=w565:bool)
        n341 = Quotient & Remainder(x=w569, y="Step size") -> (x-y*floor(x/y)=w544:dbl, floor(x/y)=w559:dbl)
        n342 = Quotient & Remainder(x=w567, y="Line displacement") -> (x-y*floor(x/y)=w556:dbl, floor(x/y)=w561:dbl)
        n343 = Less?(x=w567, y="Line displacement") -> (x < y?=w555:bool)
        n344 = Or(x=w566, y=w565) -> (x .or. y?=w558:bool)
        n345 = Or(x=w554, y=w555) -> (x .or. y?=w557:bool)
        n346 = Equal To 0?(x=w556) -> (x = 0?=w563:bool)
        n347 = Not Or(1:w557, 2:w558) -> (0:w549:bool)
        n348 = Equal To 0?(x=w544) -> (x = 0?=w564:bool)
        n349 = Select(t=1.0, s=w563, f=2.0) -> (s? t:f=w562:dbl)
        n350 = Select(t=1.0, s=w564, f=2.0) -> (s? t:f=w560:dbl)
        n351 = Add(x=w562, y=w561) -> (x+y=w575:dbl)
        n352 = Add(x=w560, y=w559) -> (x+y=w574:dbl)
        n353 = case shown="True" w549 {
          tunnel: w575 -> [_ w590]
          tunnel: w574 -> [_ w589]
          tunnel: w548 -> [_ w578]
          frame False {
          }
          frame True {
            n354 = local read "ArAy"() -> (w587:string[])
            n355 = local read "ArAx"() -> (w588:string[])
            n356 = for {
              N: w590 -> [w678]
              shift-right: [w680] -> w577
              shift-left: w587 -> [w679]
              i -> [w675]
              n357 = local read "Line displacement"() -> (w676:dbl)
              n358 = Multiply(x=w675, y=w676) -> (x*y=w668:dbl)
              n359 = Increment(x=w675) -> (x+1=w677:i32)
              n360 = local read "y1"() -> (w666:dbl)
              n361 = local read "y0"() -> (w669:dbl)
              n362 = Equal?(x=w678, y=w677) -> (x = y?=w674:bool)
              n363 = Add(x=w668, y=w669) -> (x+y=w667:dbl)
              n364 = Select(t=w666, s=w674, f=w667) -> (s? t:f=w673:dbl)
              n365 = Format Into String(format string="%#f", w673) -> (resulting string=w671:string)  [unwired: 2 in, 1 out]
              n366 = Build Array(w671) -> (w670:string[])
              n367 = Insert Into Array(array=w679, new element=w670) -> (w680:string[])  [unwired: 1 in]
            }
            n368 = for {
              N: w589 -> [w658]
              shift-right: [w665] -> w576
              shift-left: w588 -> [w664]
              i -> [w659]
              n369 = local read "Step size"() -> (w661:dbl)
              n370 = local read "x1"() -> (w651:dbl)
              n371 = Increment(x=w659) -> (x+1=w660:i32)
              n372 = local read "x0"() -> (w654:dbl)
              n373 = Multiply(x=w659, y=w661) -> (x*y=w653:dbl)
              n374 = Equal?(x=w658, y=w660) -> (x = y?=w657:bool)
              n375 = Add(x=w653, y=w654) -> (x+y=w652:dbl)
              n376 = Select(t=w651, s=w657, f=w652) -> (s? t:f=w656:dbl)
              n377 = Format Into String(format string="%#f", w656) -> (resulting string=w663:string)  [unwired: 2 in, 1 out]
              n378 = Build Array(w663) -> (w662:string[])
              n379 = Insert Into Array(array=w664, new element=w662) -> (w665:string[])  [unwired: 1 in]
            }
            n380 = Array Size(array=w577) -> (size(s)=w585:i32)
            n381 = Multiply(x="Speed (micron/s) A", y=0.06) -> (x*y=w581:dbl)
            n382 = Array Size(array=w576) -> (size(s)=w584:i32)
            n383 = Format Into String(format string="%#f", w581) -> (resulting string=w579:string)  [unwired: 2 in, 1 out]
            n384 = Reverse 1D Array(array=w576) -> (reversed array=w586:string[])
            n385 = for {
              N: w585 -> [_]
              tunnel: w576 -> [w598]
              tunnel: w586 -> [w597]
              tunnel: w584 -> [w595]
              tunnel: w577 -> [w594] mode=indexing
              tunnel: w579 -> [w593]
              tunnel: w578 -> [w592]
              i -> [w602]
              stop <- w591 stop-if-true
              n386 = Quotient & Remainder(x=w602, y=2) -> (x-y*floor(x/y)=w600:i32)  [unwired: 1 out]
              n387 = Equal To 0?(x=w600) -> (x = 0?=w599:bool)
              n388 = Select(t=w598, s=w599, f=w597) -> (s? t:f=w596:string[])
              n389 = for {
                N: w595 -> [_]
                tunnel: w596 -> [w612] mode=indexing
                tunnel: w594 -> [w613]
                tunnel: w593 -> [w615]
                tunnel: w592 -> [w614]
                tunnel: [w604] -> w591
                stop <- w604 stop-if-true
                n390 = Fract/Exp String To Number(string=w612) -> (number=w605:dbl)  [unwired: 3 in, 1 out]
                n391 = Fract/Exp String To Number(string=w613) -> (number=w606:dbl)  [unwired: 3 in, 1 out]
                n392 = Concatenate Strings("set mdi G1 X", w612, " Y" ("string"), w613, " F" ("string"), w615, "\r\n") -> (w607:string)
                n393 = flat-sequence {
                  tunnel: w614 -> [w631]
                  tunnel: [w627] -> w603
                  tunnel: w607 -> [w630]
                  tunnel: w606 -> [w635]
                  tunnel: w605 -> [w634]
                  tunnel: [w633] -> w604
                  frame #0 {
                    n394 = TCP Write(connection ID=w631, data in=w630) -> (connection ID out=w627:refnum<k5>, bytes written=w629:i32)  [unwired: 2 in, 1 out]
                    n395 = call "set_read.vi"("connection ID"=w627, "bytes to read"=w629) -> ("concatenated string"=w628:string)  [unwired: 4 in, 1 out]
                    n396 = local write "MDI"(w628) -> ()
                    "String" <- w630
                  }
                  frame #1 {
                    n397 = local write "XYXA"(TRUE ("XYXA")) -> ()
                  }
                  frame #2 {
                    n398 = while {
                      tunnel: w635 -> [w645]
                      tunnel: w634 -> [w644]
                      tunnel: ["Stop A"] -> w633
                      stop <- w638 stop-if-true
                      n399 = local read "True Y"() -> (w643:dbl)
                      n400 = local read "True X"() -> (w642:dbl)
                      n401 = Equal?(x=w643, y=w645) -> (x = y?=w640:bool)
                      n402 = Equal?(x=w642, y=w644) -> (x = y?=w641:bool)
                      n403 = And(x=w640, y=w641) -> (x .and. y?=w637:bool)
                      n404 = Or(x=w637, y="Stop A") -> (x .or. y?=w638:bool)
                      n405 = Wait (ms)(milliseconds to wait=u32 1) -> ()  [unwired: 1 out]
                    }
                  }
                  frame #3 {
                    w648 = 101.0 ("y")
                    n406 = local write "XYXA"(FALSE ("XYXA")) -> ()
                    n407 = Greater Or Equal?(x="Wait (ms) Area", y=w648) -> (x >= y?=w650:bool)
                    n408 = Select(t="Wait (ms) Area", s=w650, f=w648) -> (s? t:f=w647:dbl)
                    n409 = Wait (ms)(milliseconds to wait=w647) -> ()  [unwired: 1 out]
                  }
                }
                n410 = case shown="True" w604 {
                  tunnel: w603 -> [_ w622]
                  frame False {
                  }
                  frame True {
                    n411 = flat-sequence {
                      tunnel: ["\r\n"] -> w617
                      tunnel: ["set abort"] -> w616
                      frame #0 {
                        n412 = local write "XYXA"(FALSE ("XYXA")) -> ()
                        n413 = Wait (ms)(milliseconds to wait=u32 101) -> ()  [unwired: 1 out]
                      }
                      frame #1 {
                      }
                    }
                    n414 = Concatenate Strings(w616, w617) -> (w619:string)
                    n415 = TCP Write(connection ID=w622, data in=w619) -> (connection ID out=w621:refnum<k5>, bytes written=w620:i32)  [unwired: 2 in, 1 out]
                    n416 = call "set_read.vi"("connection ID"=w621, "bytes to read"=w620) -> ("concatenated string"=w618:string)  [unwired: 4 in, 1 out]
                    n417 = local write "MDI"(w618) -> ()
                  }
                }
              }
            }
          }
        }
      }
      frame "Enable all" {
        w681 = FALSE ("Visible")
        w683 = T14."Enabled" ("Disabled")
        w685 = T14."Enabled" ("Disabled")
        w682 = T14."Enabled" ("Disabled")
        n418 = property on="XI/YI" class="Bool (strict)"("Visible"=w681) -> ()  [unwired: 2 in, 2 out]
        n419 = property on="YV Graph" class="XYGraph (strict)"("Visible"=w681) -> ()  [unwired: 2 in, 2 out]
        n420 = property on="z-" class="Bool (strict)"("DisabledEnum"=w683) -> ()  [unwired: 2 in, 2 out]
        n421 = property on="z+" class="Bool (strict)"("DisabledEnum"=w683) -> ()  [unwired: 2 in, 2 out]
        n422 = property on="y+" class="Bool (strict)"("DisabledEnum"=w683) -> ()  [unwired: 2 in, 2 out]
        n423 = property on="x+" class="Bool (strict)"("DisabledEnum"=w683) -> ()  [unwired: 2 in, 2 out]
        n424 = property on="x-" class="Bool (strict)"("DisabledEnum"=w683) -> ()  [unwired: 2 in, 2 out]
        n425 = property on="y-" class="Bool (strict)"("DisabledEnum"=w683) -> ()  [unwired: 2 in, 2 out]
        n426 = property on="Jog?" class="Bool (strict)"("DisabledEnum"=w683) -> ()  [unwired: 2 in, 2 out]
        n427 = property on="Step size (mm)" class="DigNum (strict)"("DisabledEnum"=w683) -> ()  [unwired: 2 in, 2 out]
        n428 = property on="X0" class="DigNum (strict)"("DisabledEnum"=w682) -> ()  [unwired: 2 in, 2 out]
        n429 = property on="X1" class="DigNum (strict)"("DisabledEnum"=w682) -> ()  [unwired: 2 in, 2 out]
        n430 = property on="No. of teps" class="DigNum (strict)"("DisabledEnum"=w682) -> ()  [unwired: 2 in, 2 out]
        n431 = property on="Y0" class="DigNum (strict)"("DisabledEnum"=w682) -> ()  [unwired: 2 in, 2 out]
        n432 = property on="Y1" class="DigNum (strict)"("DisabledEnum"=w682) -> ()  [unwired: 2 in, 2 out]
        n433 = property on="Speed (micron/s) 2D" class="Knob (strict)"("DisabledEnum"=w682) -> ()  [unwired: 2 in, 2 out]
        n434 = property on="Wait (ms)" class="DigNum (strict)"("DisabledEnum"=w682) -> ()  [unwired: 2 in, 2 out]
        n435 = property on="Tab Control" class="TabCtl (strict)"("DisabledEnum"=w682) -> ()  [unwired: 2 in, 2 out]
        n436 = property on="x0" class="DigNum (strict)"("DisabledEnum"=w685) -> ()  [unwired: 2 in, 2 out]
        n437 = property on="x1" class="DigNum (strict)"("DisabledEnum"=w685) -> ()  [unwired: 2 in, 2 out]
        n438 = property on="Step size" class="DigNum (strict)"("DisabledEnum"=w685) -> ()  [unwired: 2 in, 2 out]
        n439 = property on="y0" class="DigNum (strict)"("DisabledEnum"=w685) -> ()  [unwired: 2 in, 2 out]
        n440 = property on="y1" class="DigNum (strict)"("DisabledEnum"=w685) -> ()  [unwired: 2 in, 2 out]
        n441 = property on="Line displacement" class="DigNum (strict)"("DisabledEnum"=w685) -> ()  [unwired: 2 in, 2 out]
        n442 = property on="Stop A" class="Bool (strict)"("DisabledEnum"=w685) -> ()  [unwired: 2 in, 2 out]
        n443 = property on="Speed (micron/s) A" class="Knob (strict)"("DisabledEnum"=w685) -> ()  [unwired: 2 in, 2 out]
        n444 = property on="Wait (ms) Area" class="DigNum (strict)"("DisabledEnum"=w685) -> ()  [unwired: 2 in, 2 out]
        n445 = flat-sequence {
          frame #0 {
            n446 = local write "XYXA"(TRUE ("XYXA")) -> ()
            n447 = Wait (ms)(milliseconds to wait=u32 500) -> ()  [unwired: 1 out]
          }
          frame #1 {
            w689 = FALSE ("2D stop")
            n448 = local write "2D stop"(w689) -> ()
            n449 = local write "Stop A"(w689) -> ()
            n450 = local write "Stop all"(w689) -> ()
            n451 = local write "XYXA"(w689) -> ()
            "manual" <- w689
          }
        }
      }
      frame "Move to target" {
        w691 = T14."Disabled and Grayed Out" ("Disabled")
        w692 = T14."Disabled and Grayed Out" ("Disabled")
        w690 = T14."Disabled and Grayed Out" ("Disabled")
        n452 = for {
          tunnel: w694 -> [w698] mode=indexing
          i -> [w696]
          n453 = while {
            tunnel: w698 -> [w704]
            tunnel: w696 -> [w708]
            stop <- w707 stop-if-true
            n454 = case shown="2" w708 {
              tunnel: [w709 w710 w711 w712] -> w705
              frame 0, Default {
                n455 = local read "True X"() -> (w709:dbl)
              }
              frame 1 {
                n456 = local read "True Y"() -> (w710:dbl)
              }
              frame 2 {
                n457 = local read "True Z"() -> (w711:dbl)
              }
              frame 3 {
                n458 = local read "True A"() -> (w712:dbl)
              }
            }
            n459 = Subtract(x=w705, y=w704) -> (x-y=w703:dbl)
            n460 = Absolute Value(x=w703) -> (abs(x)=w702:dbl)
            n461 = Less?(x=w702, y=0.001) -> (x < y?=w700:bool)
            n462 = local read "Stop all"() -> (w706:bool)
            n463 = Compound Arithmetic op=OR(w706, w700, "stop step") -> (w707:bool)
          }
          n464 = local write "XYXA"(TRUE ("XYXA")) -> ()
        }
        n465 = property on="X0" class="DigNum (strict)"("DisabledEnum"=w692) -> ()  [unwired: 2 in, 2 out]
        n466 = property on="X1" class="DigNum (strict)"("DisabledEnum"=w692) -> ()  [unwired: 2 in, 2 out]
        n467 = property on="Y0" class="DigNum (strict)"("DisabledEnum"=w692) -> ()  [unwired: 2 in, 2 out]
        n468 = property on="Y1" class="DigNum (strict)"("DisabledEnum"=w692) -> ()  [unwired: 2 in, 2 out]
        n469 = property on="Speed (micron/s) 2D" class="Knob (strict)"("DisabledEnum"=w692) -> ()  [unwired: 2 in, 2 out]
        n470 = property on="Wait (ms)" class="DigNum (strict)"("DisabledEnum"=w692) -> ()  [unwired: 2 in, 2 out]
        n471 = property on="No. of teps" class="DigNum (strict)"("DisabledEnum"=w692) -> ()  [unwired: 2 in, 2 out]
        n472 = property on="z-" class="Bool (strict)"("DisabledEnum"=w690) -> ()  [unwired: 2 in, 2 out]
        n473 = property on="z+" class="Bool (strict)"("DisabledEnum"=w690) -> ()  [unwired: 2 in, 2 out]
        n474 = property on="x+" class="Bool (strict)"("DisabledEnum"=w690) -> ()  [unwired: 2 in, 2 out]
        n475 = property on="Jog?" class="Bool (strict)"("DisabledEnum"=w690) -> ()  [unwired: 2 in, 2 out]
        n476 = property on="Step size (mm)" class="DigNum (strict)"("DisabledEnum"=w690) -> ()  [unwired: 2 in, 2 out]
        n477 = property on="y+" class="Bool (strict)"("DisabledEnum"=w690) -> ()  [unwired: 2 in, 2 out]
        n478 = property on="x-" class="Bool (strict)"("DisabledEnum"=w690) -> ()  [unwired: 2 in, 2 out]
        n479 = property on="y-" class="Bool (strict)"("DisabledEnum"=w690) -> ()  [unwired: 2 in, 2 out]
        n480 = property on="x0" class="DigNum (strict)"("DisabledEnum"=w691) -> ()  [unwired: 2 in, 2 out]
        n481 = property on="y0" class="DigNum (strict)"("DisabledEnum"=w691) -> ()  [unwired: 2 in, 2 out]
        n482 = property on="Step size" class="DigNum (strict)"("DisabledEnum"=w691) -> ()  [unwired: 2 in, 2 out]
        n483 = property on="Line displacement" class="DigNum (strict)"("DisabledEnum"=w691) -> ()  [unwired: 2 in, 2 out]
        n484 = property on="Wait (ms) Area" class="DigNum (strict)"("DisabledEnum"=w691) -> ()  [unwired: 2 in, 2 out]
        n485 = property on="x1" class="DigNum (strict)"("DisabledEnum"=w691) -> ()  [unwired: 2 in, 2 out]
        n486 = property on="y1" class="DigNum (strict)"("DisabledEnum"=w691) -> ()  [unwired: 2 in, 2 out]
        n487 = local read "Stop all"() -> (w695:bool)
      }
      frame "Get Values" {
      }
    }
    "main" <- w240
  }
  n488 = while {
    tunnel: w3 -> [w717]
    i -> [w719]
    stop <- w715 stop-if-true
    n489 = local read "manual"() -> (w716:bool)
    n490 = Wait (ms)(milliseconds to wait=u32 100) -> ()  [unwired: 1 out]
    n491 = case shown="True" w716 {
      tunnel: w717 -> [_ w728]
      frame False {
      }
      frame True {
        n492 = local read "Moving"() -> (w720:i32)
        n493 = Format Into String(format string="%3.3f", w720) -> (resulting string=w725:string)  [unwired: 2 in, 1 out]
        n494 = Concatenate Strings("get rel_act_pos ", w725, "\r\n") -> (w727:string)
        n495 = call "get_read.vi"("connection ID"=w728, "get command"=w727) -> ("MDI"=w722:string, "out 3DoF"=w721:dbl)  [unwired: 5 in, 2 out]
        n496 = case shown="3" w720 {
          tunnel: w721 -> [w729 w730 w731 w732]
          frame 0, Default {
            n497 = local write "True X"(w729) -> ()
          }
          frame 1 {
            n498 = local write "True Y"(w730) -> ()
          }
          frame 2 {
            n499 = local write "True Z"(w731) -> ()
          }
          frame 3 {
            n500 = local write "True A"(w732) -> ()
          }
        }
        n501 = local write "Rel_act_pos"(w722) -> ()
      }
    }
    n502 = case shown="True" "XYXA" {
      tunnel: w717 -> [_ w743]
      tunnel: w719 -> [_ w740]
      frame False {
      }
      frame True {
        n503 = Quotient & Remainder(x=w740, y=3) -> (x-y*floor(x/y)=w735:i32)  [unwired: 1 out]
        n504 = Format Into String(format string="%3.3f", w735) -> (resulting string=w738:string)  [unwired: 2 in, 1 out]
        n505 = Concatenate Strings("get rel_act_pos ", w738, "\r\n") -> (w742:string)
        n506 = call "get_read.vi"("connection ID"=w743, "get command"=w742) -> ("MDI"=→"Rel_act_pos":string, "out 3DoF"=w734:dbl)  [unwired: 5 in, 2 out]
        n507 = case shown="3" w735 {
          tunnel: w734 -> [w744 w745 w746 w747]
          frame 0, Default {
            "True X" <- w744
          }
          frame 1 {
            "True Y" <- w745
          }
          frame 2 {
            "True Z" <- w746
          }
          frame 3 {
            "True A" <- w747
          }
        }
      }
    }
    n508 = local read "Stop all"() -> (w715:bool)
    "position" <- w715
  }
  n509 = property on="Rel_act_pos" class="Str"("Visible"=w2) -> ()  [unwired: 2 in, 2 out]
  n510 = property on="ArAx" class="Arr (strict)"("Visible"=w2) -> ()  [unwired: 2 in, 2 out]
  n511 = property on="Iarray" class="Arr (strict)"("Visible"=w2) -> ()  [unwired: 2 in, 2 out]
  n512 = property on="Curves" class="Arr (strict)"("Visible"=w2) -> ()  [unwired: 2 in, 2 out]
  n513 = property on="Yarray" class="Arr (strict)"("Visible"=w2) -> ()  [unwired: 2 in, 2 out]
  n514 = property on="Status" class="Bool (strict)"("Visible"=w2) -> ()  [unwired: 2 in, 2 out]
  n515 = property on="ArAy" class="Arr (strict)"("Visible"=w2) -> ()  [unwired: 2 in, 2 out]
  n516 = property on="Xarray" class="Arr (strict)"("Visible"=w2) -> ()  [unwired: 2 in, 2 out]
  n517 = property on="Moving" class="DigNum (strict)"("Visible"=w1) -> ()  [unwired: 2 in, 2 out]
  n518 = property on="Serial Settings" class="Clust (strict)"("Visible"=w1) -> ()  [unwired: 2 in, 2 out]
  n519 = property on="Node list" class="Tree (strict)"("Visible"=w1) -> ()  [unwired: 2 in, 2 out]
  n520 = property on="main" class="Bool (strict)"("Visible"=w1) -> ()  [unwired: 2 in, 2 out]
  n521 = property on="potentiostat" class="Bool (strict)"("Visible"=w1) -> ()  [unwired: 2 in, 2 out]
  n522 = property on="Camera" class="Bool (strict)"("Visible"=w1) -> ()  [unwired: 2 in, 2 out]
  n523 = property on="graphs" class="Bool (strict)"("Visible"=w1) -> ()  [unwired: 2 in, 2 out]
  n524 = property on="position" class="Bool (strict)"("Visible"=w1) -> ()  [unwired: 2 in, 2 out]
  n525 = property on="Cluster" class="Clust (strict)"("Visible"=w5) -> ()  [unwired: 2 in, 2 out]
  n526 = property on="Cluster 2" class="Clust (strict)"("Visible"=w5) -> ()  [unwired: 2 in, 2 out]
  n527 = property on="Cluster 3" class="Clust (strict)"("Visible"=w5) -> ()  [unwired: 2 in, 2 out]
  n528 = property on="Cluster 4" class="Clust (strict)"("Visible"=w5) -> ()  [unwired: 2 in, 2 out]
  n529 = property on="Cluster 5" class="Clust (strict)"("Visible"=w5) -> ()  [unwired: 2 in, 2 out]
  "MDI" <- w32
